vi "main 1.1 stable.vi"() -> ()   [LabVIEW 2020]
uses:
  subvi/Newport ESP301/Newport ESP301.lvlib
  subvi/sp_manip.llb/sp_manip_lib.lvlib
  subvi/sp_manip.llb/tcp_gateway.lvlib
  subvi/PHOIBOS/DEFINITIONS/DEF_dev_type.ctl
  subvi/PHOIBOS/DEFINITIONS/DEF_dev_state.ctl
  <vilib>/Utility/file.llb/Write Delimited Spreadsheet (DBL).vi
  <vilib>/Analysis/NI_AALBase.lvlib
  <vilib>/Analysis/1siggen.llb/Ramp Pattern by Samples.vi
  <vilib>/Analysis/NI_AALPro.lvlib
  <vilib>/Analysis/_algsub.llb/Real Vector Norm.vi
  subvi/ZaberTSeries/ZaberTSeries.lvlib
  <vilib>/DAQmx/create/channels.llb/DAQmx Create Channel (DI-Digital Input).vi
  <vilib>/Utility/file.llb/Read Delimited Spreadsheet (string).vi
  <vilib>/Utility/file.llb/Write Delimited Spreadsheet (string).vi
panel:
  out "Pics L":i32=20
  out "Waveform Chart":dbl(graph)
  out "G2 X":cluster{dbl[], "Ramp Pattern":dbl[]}(graph)
  in  "reset every n pics":bool=TRUE
  in  "pics2avg":i32=50
  in  "abort acq.":bool
  out "G2 Y":cluster{dbl[], "Ramp Pattern":dbl[]}(graph)={[0.0, 0.0, 0.0, 0.0, 0.0, 0.0, 0.0, 0.0, 0.0, 0.0, 0.0, 0.0, 0.0, 0.0, 0.0, 0.0, 0.0, 0.0, 0.0, 0.0, 0.0, 0.0, 0.0, 0.0, 0.0, 0.0, 0.0, 0.0, 0.0, 0.0, 0.0, 0.0, 0.0, 0.0, 0.0, 0.0, 0.0, 0.0, 0.0, 0.0, 0.0, 0.0, 0.0, 0.0, 0.0, 0.0, 0.0, 0.0, 0.0, 0.0, 0.0, 0.0, 0.0, 0.0, 0.0, 0.0, 0.0, 0.0, 0.0, 0.0, 0.0, 0.0, 0.0, 0.0, 0.0, 0.0, 0.0, 0.0, 0.0, 0.0, 0.0, 0.0, 0.0, 0.0, 0.0, 0.0, 0.0, 0.0, 0.0, 0.0, 0.0, 0.0, 0.0, 0.0, 0.0, 0.0, 0.0, 0.0, 0.0, 0.0, 0.0, 0.0, 0.0, 0.0, 0.0, 0.0, 0.0, 0.0, 0.0, 0.0, 0.0, 0.0, 0.0, 0.0, 0.0, 0.0, 0.0, 0.0, 0.0, 0.0, 0.0, 0.0, 0.0, 0.0, 0.0, 0.0, 0.0, 0.0, 0.0, 0.0, 0.0, 0.0, 0.0, 0.0, 0.0, 0.0, 0.0, 0.0, 0.0, 0.0, 0.0, 0.0, 0.0, 0.0, 0.0, 0.0, 0.0, 0.0, 0.0, 0.0, 0.0, 0.0, 0.0, 0.0, 0.0, 0.0, 0.0, 0.0, 0.0, 0.0, 0.0, 0.0, 0.0, 0.0, 0.0, 0.0, 0.0, 0.0, 0.0, 0.0, 0.0, 0.0, 0.0, 0.0, 0.0, 0.0, 0.0, 0.0, 0.0, 0.0, 0.0, 0.0, 0.0, 0.0, 0.0, 0.0, 0.0, 0.0, 0.0, 0.0, 0.0, 0.0, 0.0, 0.0, 0.0, 0.0, 0.0, 0.0, 0.0, 0.0, 0.0, 0.0, 0.0, 0.0, 0.0, 0.0, 0.0, 0.0, 0.0, 0.0, 0.0, 0.0, 0.0, 0.0, 0.0, 0.0, 0.0, 0.0, 0.0, 0.0, 0.0, 0.0, 0.0, 0.0, 0.0, 0.0, 0.0, 0.0, 0.0, 0.0, 0.0, 0.0, 0.0, 0.0, 0.0, 0.0, 0.0, 0.0, 0.0, 0.0, 0.0, 0.0, 0.0, 0.0, 0.0, 0.0, 0.0, 0.0, 0.0, 0.0, 0.0, 0.0, 0.0, 0.0, 0.0, 0.0, 0.0, 0.0, 0.0, 0.0, 0.0, 0.0, 0.0, 0.0, 0.0, 0.0], "Ramp Pattern"=[0.0, 1.003921568627451, 2.007843137254902, 3.011764705882353, 4.015686274509804, 5.019607843137255, 6.023529411764706, 7.027450980392157, 8.031372549019608, 9.035294117647059, 10.03921568627451, 11.04313725490196, 12.047058823529412, 13.050980392156863, 14.054901960784314, 15.058823529411764, 16.062745098039215, 17.066666666666666, 18.070588235294117, 19.07450980392157, 20.07843137254902, 21.08235294117647, 22.08627450980392, 23.090196078431372, 24.094117647058823, 25.098039215686274, 26.101960784313725, 27.105882352941176, 28.109803921568627, 29.113725490196078, 30.11764705882353, 31.12156862745098, 32.12549019607843, 33.129411764705885, 34.13333333333333, 35.13725490196079, 36.141176470588235, 37.14509803921569, 38.14901960784314, 39.15294117647059, 40.15686274509804, 41.16078431372549, 42.16470588235294, 43.168627450980395, 44.17254901960784, 45.1764705882353, 46.180392156862744, 47.1843137254902, 48.188235294117646, 49.1921568627451, 50.19607843137255, 51.2, 52.20392156862745, 53.207843137254905, 54.21176470588235, 55.21568627450981, 56.219607843137254, 57.22352941176471, 58.227450980392156, 59.23137254901961, 60.23529411764706, 61.23921568627451, 62.24313725490196, 63.247058823529414, 64.25098039215686, 65.25490196078431, 66.25882352941177, 67.26274509803922, 68.26666666666667, 69.27058823529411, 70.27450980392157, 71.27843137254902, 72.28235294117647, 73.28627450980392, 74.29019607843138, 75.29411764705883, 76.29803921568627, 77.30196078431372, 78.30588235294118, 79.30980392156863, 80.31372549019608, 81.31764705882352, 82.32156862745099, 83.32549019607843, 84.32941176470588, 85.33333333333333, 86.33725490196079, 87.34117647058824, 88.34509803921569, 89.34901960784313, 90.3529411764706, 91.35686274509804, 92.36078431372549, 93.36470588235294, 94.3686274509804, 95.37254901960785, 96.37647058823529, 97.38039215686274, 98.3843137254902, 99.38823529411765, 100.3921568627451, 101.39607843137254, 102.4, 103.40392156862745, 104.4078431372549, 105.41176470588235, 106.41568627450981, 107.41960784313726, 108.4235294117647, 109.42745098039215, 110.43137254901961, 111.43529411764706, 112.43921568627451, 113.44313725490196, 114.44705882352942, 115.45098039215686, 116.45490196078431, 117.45882352941176, 118.46274509803922, 119.46666666666667, 120.47058823529412, 121.47450980392156, 122.47843137254903, 123.48235294117647, 124.48627450980392, 125.49019607843137, 126.49411764705883, 127.49803921568628, 128.50196078431372, 129.50588235294117, 130.50980392156862, 131.51372549019607, 132.51764705882354, 133.521568627451, 134.52549019607844, 135.52941176470588, 136.53333333333333, 137.53725490196078, 138.54117647058823, 139.54509803921567, 140.54901960784315, 141.5529411764706, 142.55686274509804, 143.5607843137255, 144.56470588235294, 145.5686274509804, 146.57254901960783, 147.57647058823528, 148.58039215686276, 149.5843137254902, 150.58823529411765, 151.5921568627451, 152.59607843137255, 153.6, 154.60392156862744, 155.6078431372549, 156.61176470588236, 157.6156862745098, 158.61960784313726, 159.6235294117647, 160.62745098039215, 161.6313725490196, 162.63529411764705, 163.6392156862745, 164.64313725490197, 165.64705882352942, 166.65098039215687, 167.65490196078431, 168.65882352941176, 169.6627450980392, 170.66666666666666, 171.6705882352941, 172.67450980392158, 173.67843137254903, 174.68235294117648, 175.68627450980392, 176.69019607843137, 177.69411764705882, 178.69803921568626, 179.7019607843137, 180.7058823529412, 181.70980392156864, 182.71372549019608, 183.71764705882353, 184.72156862745098, 185.72549019607843, 186.72941176470587, 187.73333333333332, 188.7372549019608, 189.74117647058824, 190.7450980392157, 191.74901960784314, 192.75294117647059, 193.75686274509803, 194.76078431372548, 195.76470588235293, 196.7686274509804, 197.77254901960785, 198.7764705882353, 199.78039215686275, 200.7843137254902, 201.78823529411764, 202.7921568627451, 203.79607843137254, 204.8, 205.80392156862746, 206.8078431372549, 207.81176470588235, 208.8156862745098, 209.81960784313725, 210.8235294117647, 211.82745098039214, 212.83137254901962, 213.83529411764707, 214.8392156862745, 215.84313725490196, 216.8470588235294, 217.85098039215686, 218.8549019607843, 219.85882352941175, 220.86274509803923, 221.86666666666667, 222.87058823529412, 223.87450980392157, 224.87843137254902, 225.88235294117646, 226.8862745098039, 227.89019607843136, 228.89411764705883, 229.89803921568628, 230.90196078431373, 231.90588235294118, 232.90980392156862, 233.91372549019607, 234.91764705882352, 235.92156862745097, 236.92549019607844, 237.9294117647059, 238.93333333333334, 239.93725490196078, 240.94117647058823, 241.94509803921568, 242.94901960784313, 243.95294117647057, 244.95686274509805, 245.9607843137255, 246.96470588235294, 247.9686274509804, 248.97254901960784, 249.9764705882353, 250.98039215686273, 251.98431372549018, 252.98823529411766, 253.9921568627451, 254.99607843137255, 256.0]}
  out "ETA":timestamp=timestamp(3553173084.423481 s since 1904-01-01) format="%<%H:%M:%S>T"
  out "acq. imgs":i32=20
  out "snap_prog":dbl(slide)=1.0 scale=0.0..1.0
  in  "BasePath":path=path "Z:/PESdata"
  in  "cam_liveavg":bool=TRUE caption="live average"
  out "cam_fps":dbl=19.770971874875205 caption="FPS" format="%.1g"
  out "sideimg":dbl[][](graph)
  out "RunNumber":u16=50
  out "sum":dbl format="%#.2g"
  out "max":dbl
  out "mainimg":dbl[][](graph)
  out "ESP_con?":bool=TRUE caption="ESP301"
  out "phoib_con?":bool caption="PHOIBOS"
  out "manip_con?":bool=TRUE caption="manipulator"
  out "cam_con?":bool caption="camera"
  in  "main_close":bool
  in  "Tab Control":enum32{"live", "1D scan", "devices"}(tab)=enum."1D scan"
  in  "mirr_go":bool
  in  "ESP_opent0file":bool
  in  "mirr_rel":i32=20 caption="relative [steps]"
  in  "mirr_Y-":bool
  in  "mirr_Y+":bool
  in  "mirr_X+":bool
  in  "mirr_X-":bool
  in  "manip_deltas":dbl[](array[numeric])=[0.0, 0.0, 5.0, 0.0, 0.0, 0.0] caption="delta" format="%#.5g"
  in  "aq.mode":enum32{"Radio Selection 1", "Radio Selection 2"}(radio)=enum."Radio Selection 2"
  in  "dark avg":i32=100
  in  "cam_avgs":i32=20 caption="N"
  in  "ESP_delta":dbl caption="relative [mm]"
  in  "ESP_-":bool
  in  "ESP_+":bool
  in  "ESP_go":bool
  in  "ESP_dest_t":dbl=-12656.75602819869 caption="[fs]"
  in  "ESP_dest":dbl=25.0 caption="[mm]"
  in  "ESP_set_t0":bool
  in  "phoib_I_6s":dbl=3200.0
  in  "phoib_I_5s":dbl=1500.0
  in  "phoib_I_4s":dbl=4.558
  in  "phoib_I_3s":dbl=-7.0
  in  "phoib_I_2s":dbl=30.0
  in  "phoib_I_1s":dbl=18.0
  in  "phoib_standby":bool
  in  "phoib_set":bool
  out "phoib_I_6":dbl caption="Screen Voltage"
  out "phoib_I_5":dbl caption="Detctor Voltage"
  out "phoib_I_4":dbl caption="Work Function"
  out "phoib_I_3":dbl caption="Coil Current"
  out "phoib_I_2":dbl caption="Pass Energy"
  out "phoib_I_1":dbl caption="Kinetic Energy"
  out "Saved Positions":string[][](table)=[["ertwertwert", "-2.299945", "-2.030214", "38.900024", "50.000762", "0.000887", "-97.998082"], ["uztgugt", "-14.999451", "-13.638894", "442.380066", "13.998380", "-1.893758", "-76.305838"], ["asdf", "-14.999451", "-13.638894", "442.380066", "13.998380", "-1.893758", "-76.305838"], ["test3", "-14.999451", "-13.638894", "441.380066", "13.998380", "-1.893758", "-76.305838"]]
  in  "Save Pos":bool
  in  "Load":bool
  in  "Delete":bool
  in  "ManipRel +":bool
  in  "ManipRel -":bool
  in  "Move Abs":bool
  in  "stop manip":bool
  in  "dest":dbl[](array[numeric])=[-2.599774415331921, 2.6001372083008483, 64.7374267578125, 44.999124169862, 0.0008789063100814859, -80.99718876558107] caption="destination" format="%#.5g"
  out "axis":string[](array[string])=["x", "y", "z", "polar", "tilt", "azimut"]
  out "pos":dbl[](array[numeric])=[-1.8981328134268227, 1.9037561044451934, 84.7381591796875, 38.14189713860625, 0.0008789063100814859, -70.9987511093555] caption="position" format="%.5f"
  in  "ana_mode":T1(ring)=enum."WideAngleMode"
  in  "ana_voltrange":enum16{"3.5kV", "1.5kV", "400V", "100V", "10V"}(ring)=enum."400V"
  out "ESP_pos":dbl=31.74535 caption="Position"
  out "ESP_delay":dbl=45000.131390897084 caption="Delay"
  out "ESP_t0":dbl=25.0 caption="Time Zero @"
  out "phoib_I_7":dbl caption="Conversion Voltage"
  in  "phoib_I_7s":dbl=-26.0
  in  "phoib_I_8s":dbl=0.0039
  in  "phoib_I_9s":dbl=0.0039
  out "phoib_I_8":dbl caption="FD1"
  out "phoib_I_9":dbl caption="FD2"
  in  "gain":bool
  in  "cam_exp":u32=50 caption="exposure [ms]"
  in  "binning":u16(ring)=2 items=["X 1", "X 2", "X 4", "X 8"]
  in  "cam_dark?":bool=TRUE caption="subtract dark?"
  in  "cam_dark":bool
  in  "cam_saveimg":bool
  in  "e-size":u8
  in  "lower threshold":i32=50
  in  "count?":bool
  in  "ROI Left":i32=1
  in  "ROI Right":i32=43
  in  "ROI Top":i32=1
  in  "ROI Bottom":i32=33
  out "moving?":bool[](array[boolean])
  out "mirr_posX":i32=-9907 caption="X"
  out "mirr_posY":i32=-7260 caption="Y"
  in  "mirr_dest":i32[](array[numeric])=[-64, -2601]
  out "anglegraph":dbl[][](graph)
  out "intensitygraph":cluster{"Array":dbl[], "Intensity Chart":dbl[]}(graph)={"Array"=[-100000.0, -95000.0, -90000.0, -85000.0, -80000.0, -75000.0, -70000.0, -65000.0, -60000.0, -55000.0, -50000.0, -45000.0, -40000.0, -35000.0, -30000.0, -25000.0, -20000.0, -15000.0, -10000.0, -5000.0, 0.0, 5000.0, 10000.0, 15000.0, 20000.0, 25000.0, 30000.0, 35000.0, 40000.0, 45000.0, 50000.0], "Intensity Chart"=[710968.0999999978, 661453.8299999974, 660491.1499999983, 654490.9100000008, 607000.039999999, 668861.0999999981, 631366.7699999984, 739689.6549999982, 681310.9099999986, 658872.4599999987, 692812.8950000014, 671304.7250000003, 670701.9799999978, 684100.4049999971, 706126.3150000001, 744782.0600000009, 684440.8499999981, 704157.155, 756957.4599999988, 768506.4449999956, 761428.5800000022, 678039.9949999974, 735774.9649999988, 659533.465000001, 724648.9199999974, 705546.0750000002, 773026.2399999972, 698578.0149999986, 697856.3899999985, 787613.0450000013, 750231.4800000007]}
  in  "scan_selector":enum32{"delay", "manip", "mirror", "volt"}(tab)
  in  "scan_manip_setstart":bool
  in  "scan_manip_start":dbl[](array[numeric])=[-2.6172862113166087, -0.009888298846365134, 68.5008544921875, -46.363686276590336, 11.108982061941884, -218.56360350415366] caption="start position" format="%#.5g"
  in  "scan_manip_deltas":dbl[](array[numeric])=[0.0, 0.0, 0.0, 0.0, 10.0, 0.0] caption="direction vector\n(gets normed)" format="%#.5g"
  in  "scan_mirr_start":i32[](array[numeric])=[-64, -2601]
  in  "scan_mirr_deltas":i32[](array[numeric])=[0, 0, 0, 0, 10, 0] caption="direction vector\n(gets normed)"
  in  "scan_mirr_setstart":bool
  in  "scan_volt_parameter":string(combo)="Kinetic Energy"
  in  "meas_iter":i32=60 caption="Iterations"
  out "duration [HH:MM:SS]":dbl=4512.494100093842 format="%<%H:%M:%S>t"
  out "disk [MB]":dbl=1028.5800000000002
  out "RAM [MB]":dbl=17.143
  out "total steps":i32=1860
  out "measpoints":i32=31
  in  "load delay table":bool
  in  "scan_go":bool
  in  "waypoints":string[][](table)=[["-100000", "5000"], ["50000", ""], ["", ""]]
  in  "stop after step":bool
  out "scan":dbl(slide)=0.967741935483871 scale=0.0..1.0
  out "iteration":dbl(slide)=0.03333333333333333 scale=0.0..1.0
  out "current scan":i32=30
  out "current iteration":i32=2
  in  "time/step [s]":dbl=2.426072096824646
  in  "stop after iteration":bool
  out "energygraph":dbl[][](graph)
  in  "mirr_init":bool
  in  "mirr_release":bool
  in  "mirr_Y#":u8=2
  in  "manip_init":bool
  in  "manip_release":bool
  in  "phoib_init":bool
  in  "phoib_release":bool
  in  "ESP_init":bool
  in  "ESP_release":bool
  in  "ESP301 VISA":refnum<visa-resource-name>="COM8"
  in  "board number":i32
  in  "cam_init":bool
  in  "cam_release":bool
  out "cam_error":errorcluster
  out "phoib_error":errorcluster
  out "state":T2 items=["Off"=-1, "Standby"=0, "On"=1]
  in  "ESP Axis":i32=1 min=1 max=3
  out "error out":errorcluster
  out "error out 2":errorcluster
  out "mirr_Error":errorcluster
  in  "mirr_VISA":refnum<visa-resource-name>="COM7"
  in  "mirr_X#":u8=1
  in  "Operating mode\nHP & QE / HS & DiCam Pro":u32=1
  in  "Frame trigger \n(High Performance and QE only)":u16
  # "camera"
  # "analyzer"
  # "manipulator"
  # "aquisition"
  # "delay stage"
  # "mirror"
  # "Position"
  # "Destination"
  # "- no settings -"
  # "waypoints are absolute values"
  # "X\nY\nZ\npolar\ntilt\nazimut"
  # "waypoint \"0\" is start position"
  # "X\nY"
  # "waypoint \"0\" is start position"
  # "waypoints are absolute values"
  # "camera"
  # "phoibos"
  # "ESP301"
  # "manipulator"
  # "mirror"
  # "0 = sequential\n1 = simultaneous"
  # "0 = internal\n1 = external rising\n2 = external falling"
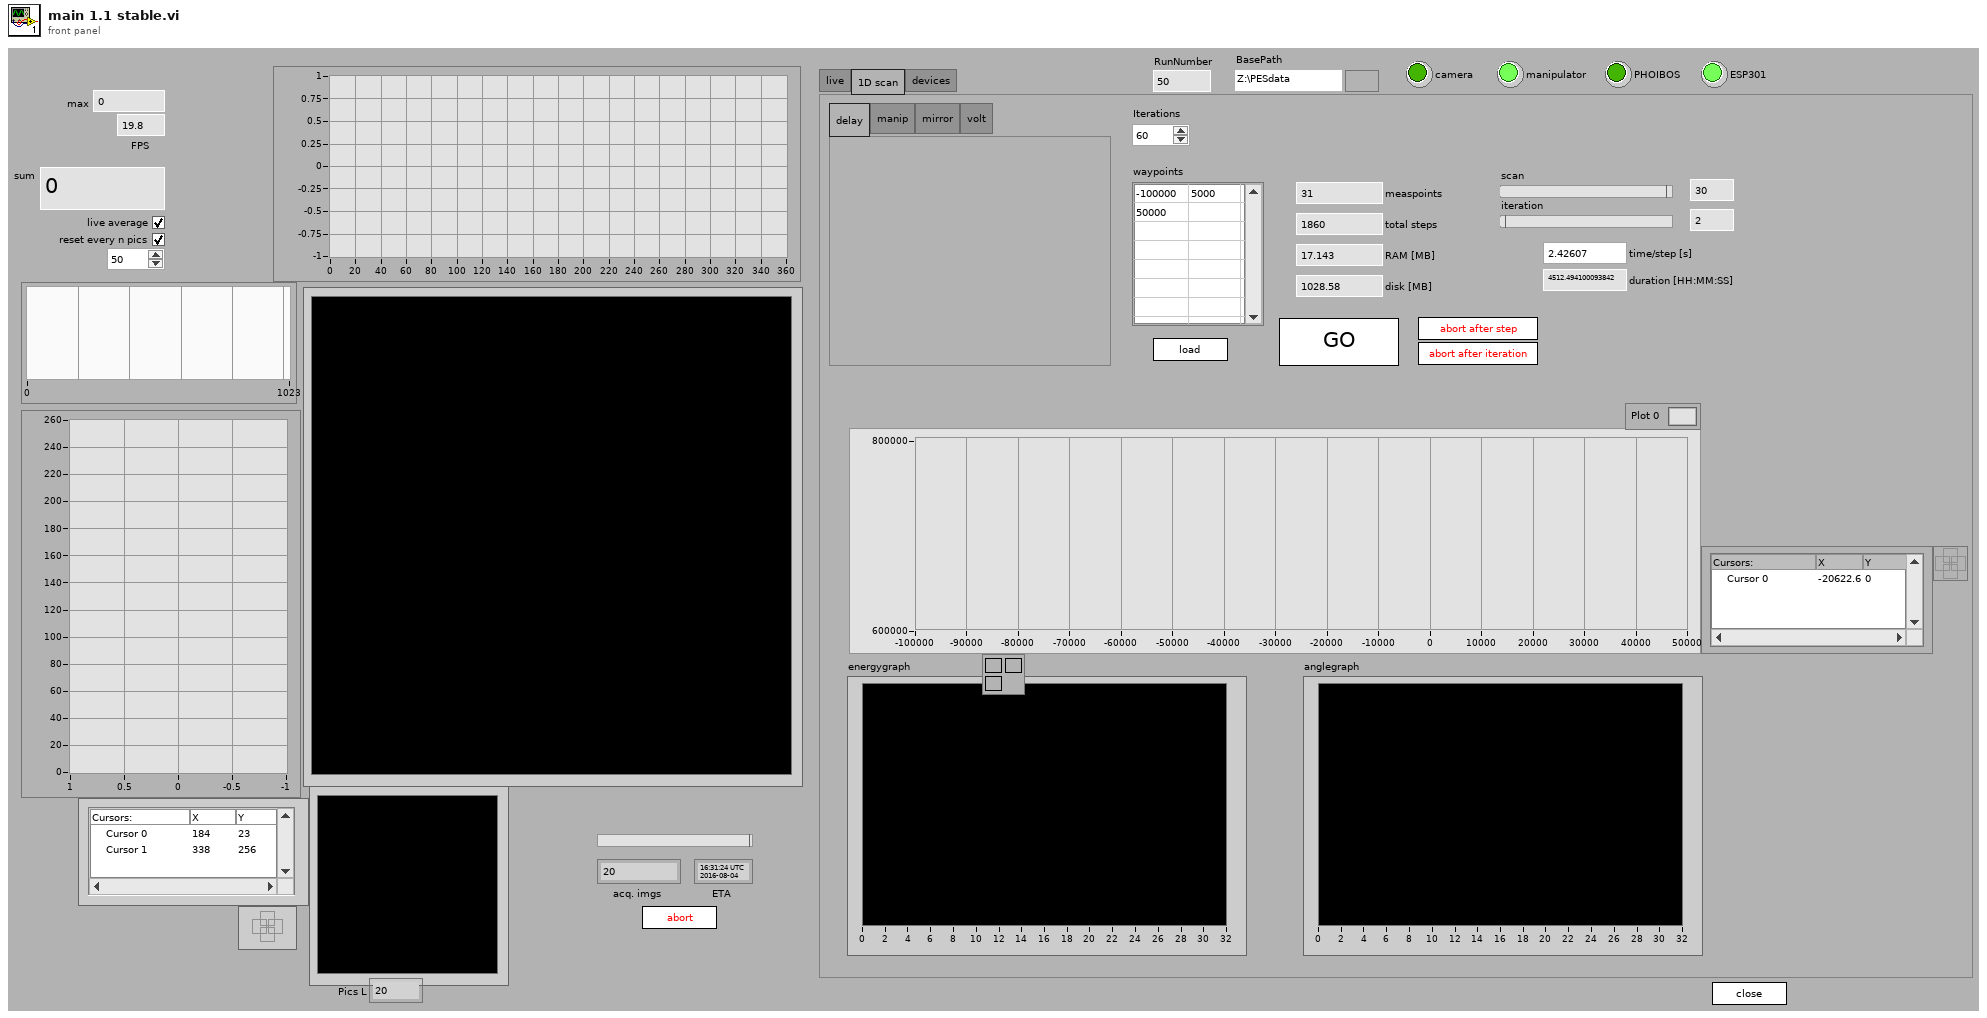
[diagram p1: front panel]
types:
  T1 = enum16{"HighMagnification", "MediumMagnification", "LowMagnification", "HighAngularDispersion", "MediumAngularDispersion", "LowAngularDispersion", "WideAngleMode", "LargeArea", "MediumArea", "SmallArea", "HighMagnification2", "SmallArea2", "ImagingMode"}
  T2 = typedef "DEF_dev_state.ctl" = i32
  T3 = cluster{"queue out":refnum<queue>, "queue out":refnum<queue>, "queue out":refnum<queue>, "queue out":refnum<queue>, "queue out":refnum<queue>}
  T4 = typedef "LVCursorListTypeDef.ctl" = cluster{"Name":string, "Color":u32, "Style":u8, "Point Style":u8, "Name Visible":bool, "Allow Drag":bool, "Cursor Mode":u32, "Plot":i32, "Index":i32, "Position":cluster{"X":dbl, "Y":dbl}, "X Scale":u32, "Y Scale":u32, "Watch Plots":i32[], "Watch All Plots":bool, "Plot Area":i32, "Label Offset":cluster{"X":dbl, "Y":dbl}}[]
  T5 = cluster{"Camera type":u32, "Operating mode\nHP & QE / HS & DiCam Pro ":u32, "Frame trigger \n(High Performance and QE only)":u16, "Sequence trigger":u16, "Low Light\n(QE only)":bool, "Gain":bool, "Horzontal\nbinning":u16, "Vertical\nbinning ":u16, "ROI Left":i32, "ROI Right":i32, "ROI Top":i32, "ROI Bottom":i32}
  T6 = cluster{"Name":string, "Color":u32, "Style":u8, "Point Style":u8, "Name Visible":bool, "Allow Drag":bool, "Cursor Mode":u32, "Plot":i32, "Index":i32, "Position":cluster{"X":dbl, "Y":dbl}, "X Scale":u32, "Y Scale":u32, "Watch Plots":i32[], "Watch All Plots":bool, "Plot Area":i32, "Label Offset":cluster{"X":dbl, "Y":dbl}}
  T7 = cluster{"mirr_X#":u8, "Command":u8, dbl, "Response Count":i32}
  T8 = cluster{"mirr_Y#":u8, "Command":u8, dbl, "Response Count":i32}
  T9 = cluster{i32, "Command":u8, i32, "Response Count":i32}
  T10 = cluster{"Axis_Name":string, "Axis_Type":string, "Axis_Position":dbl, "continous":bool, "moving":bool}[]
  T11 = typedef "DEF_dev_type.ctl" = enum32{"devA (analyzer)", "devD (detector)"}
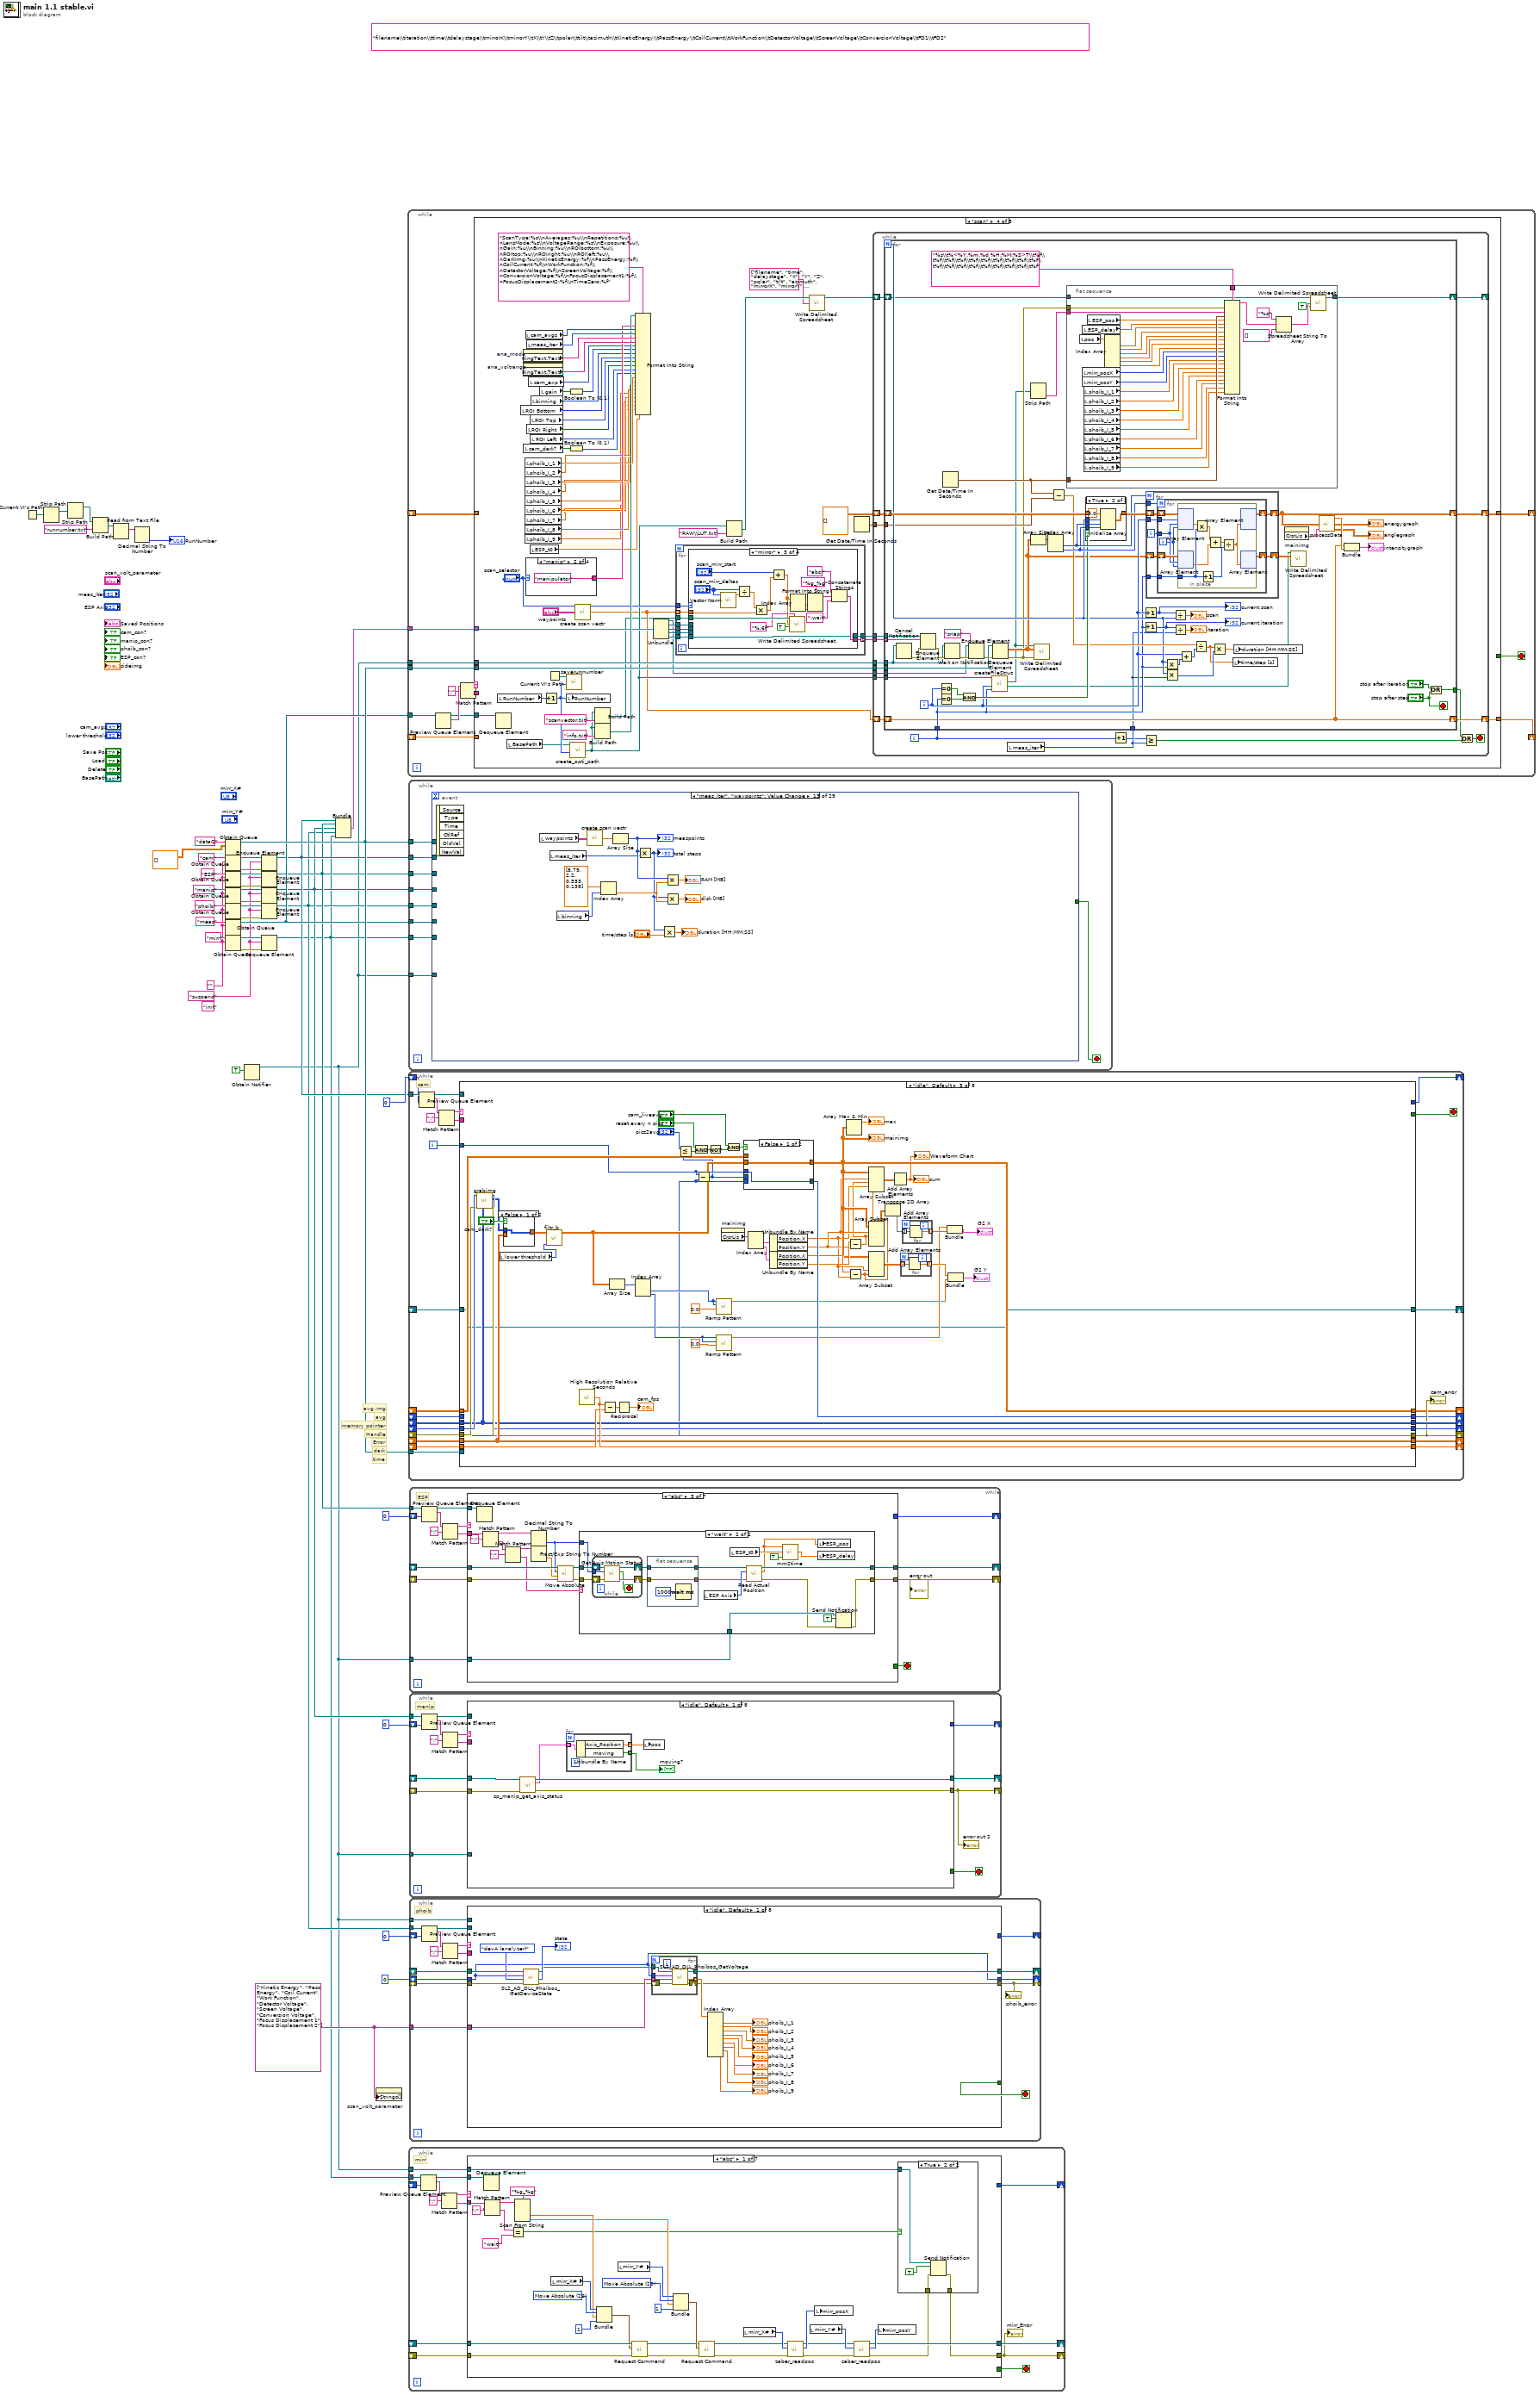
[diagram p0: block diagram]
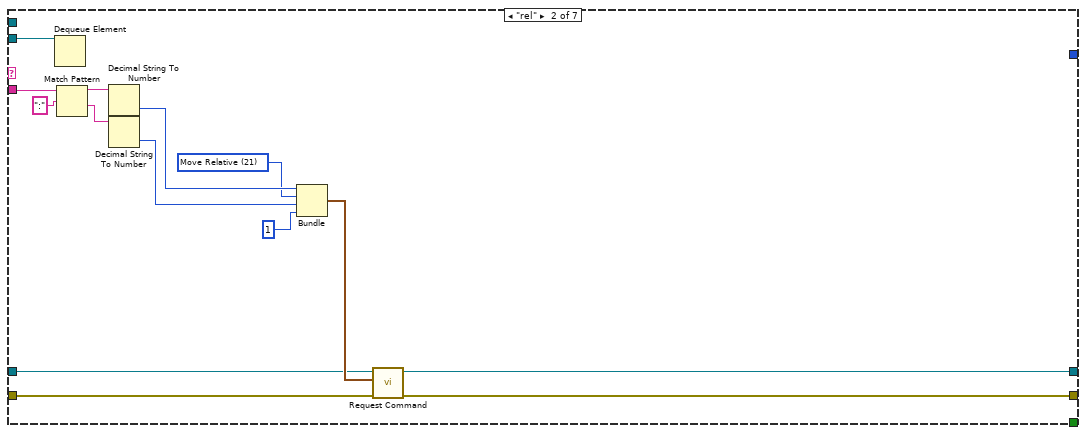
[diagram p3: hidden frame]
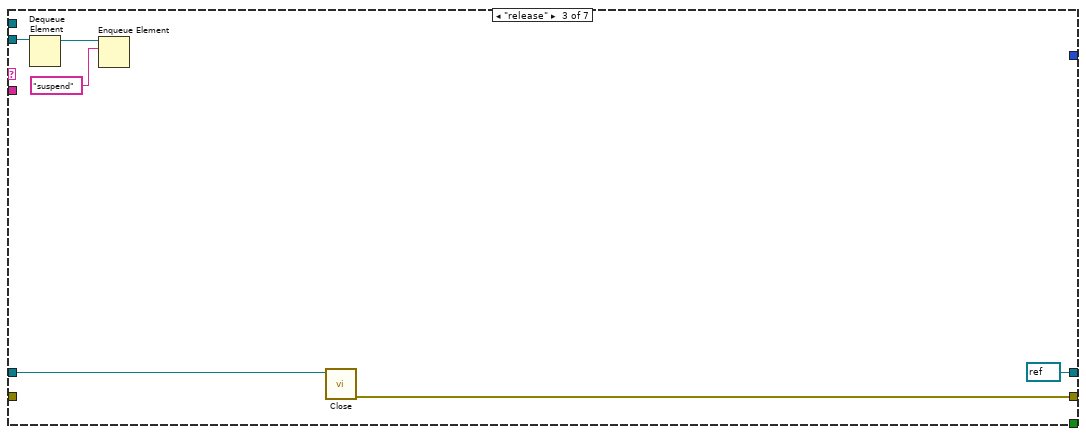
[diagram p4: hidden frame]
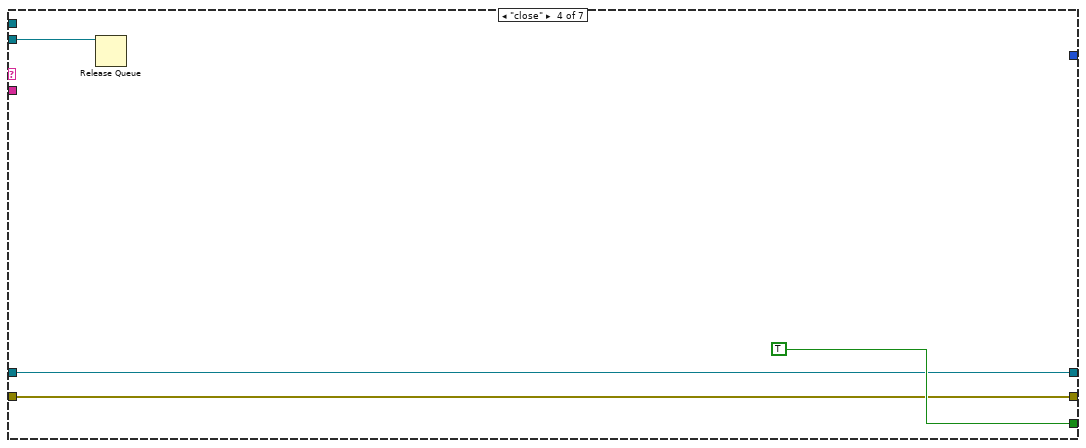
[diagram p5: hidden frame]
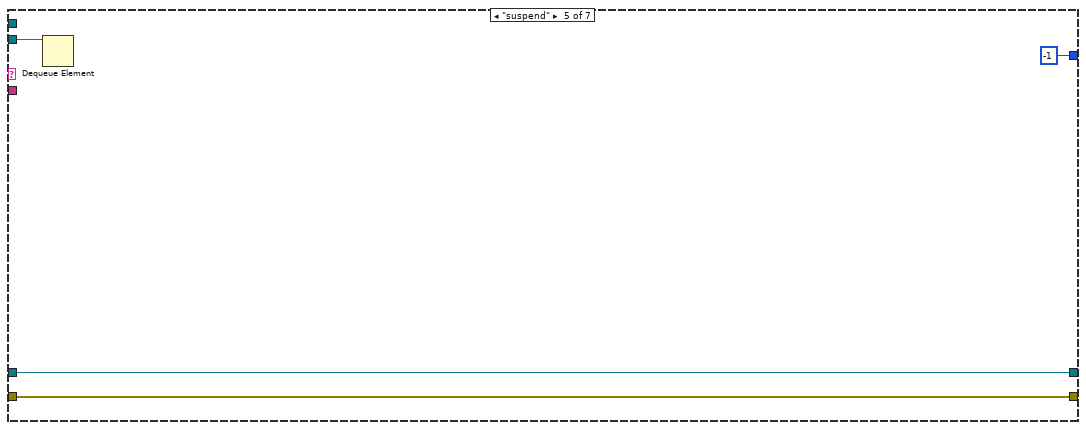
[diagram p6: hidden frame]
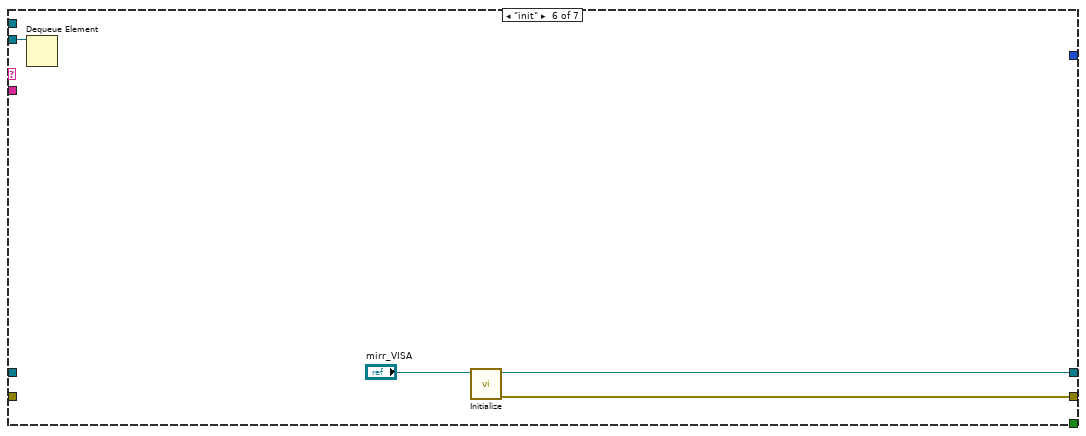
[diagram p7: hidden frame]
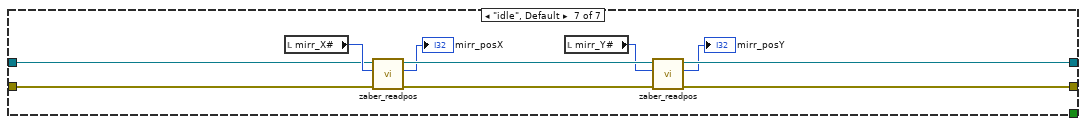
[diagram p8: hidden frame]
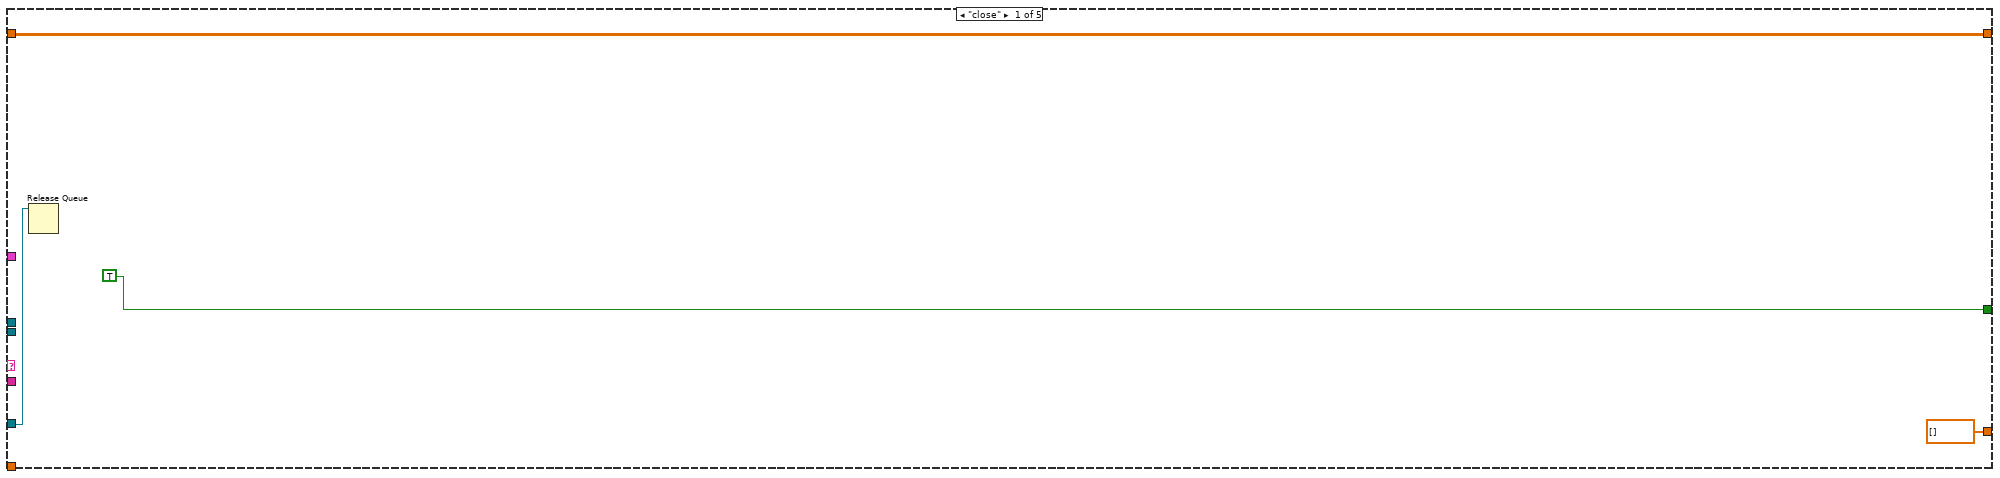
[diagram p9: hidden frame]
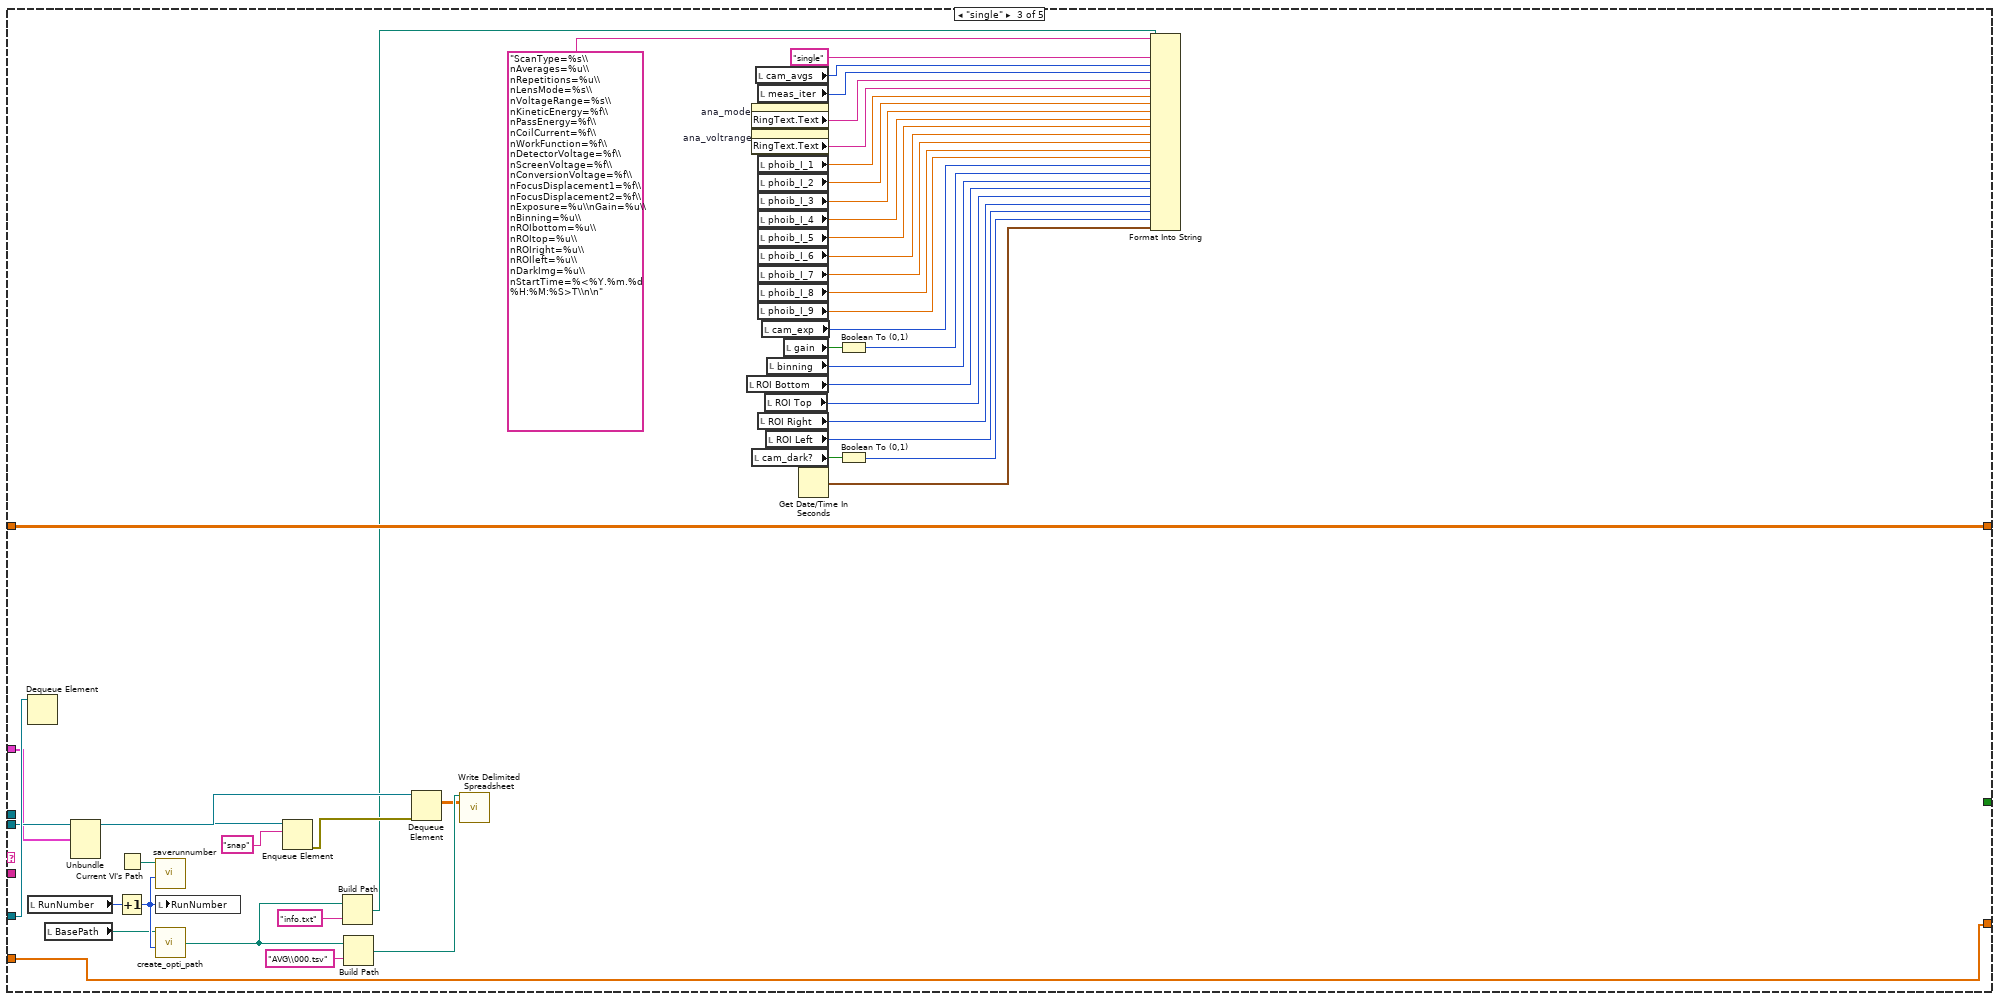
[diagram p11: hidden frame]
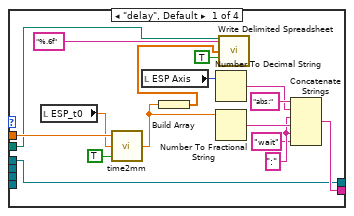
[diagram p13: hidden frame]
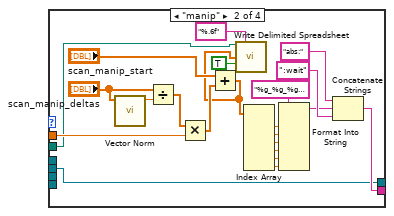
[diagram p14: hidden frame]
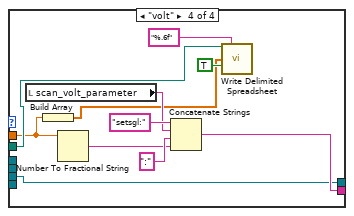
[diagram p15: hidden frame]
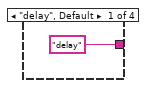
[diagram p16: hidden frame]
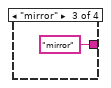
[diagram p17: hidden frame]
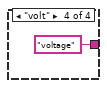
[diagram p18: hidden frame]
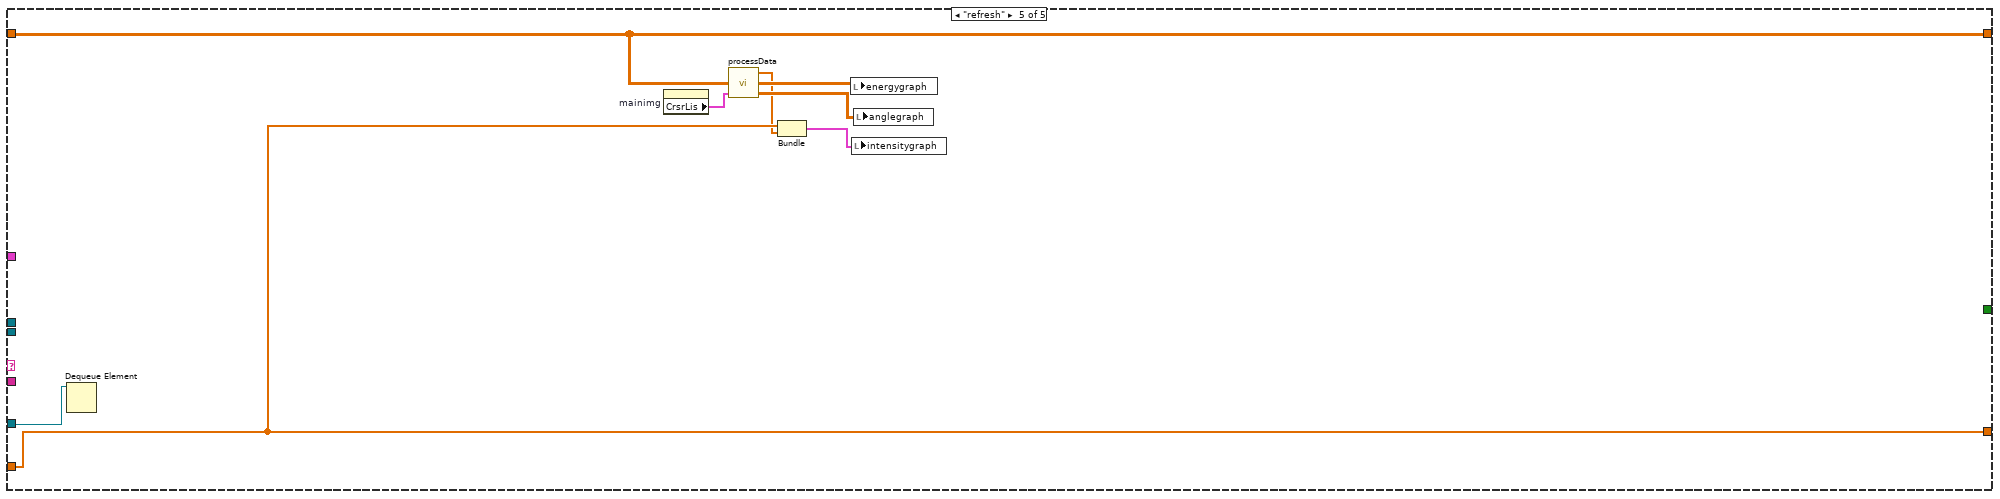
[diagram p19: hidden frame]
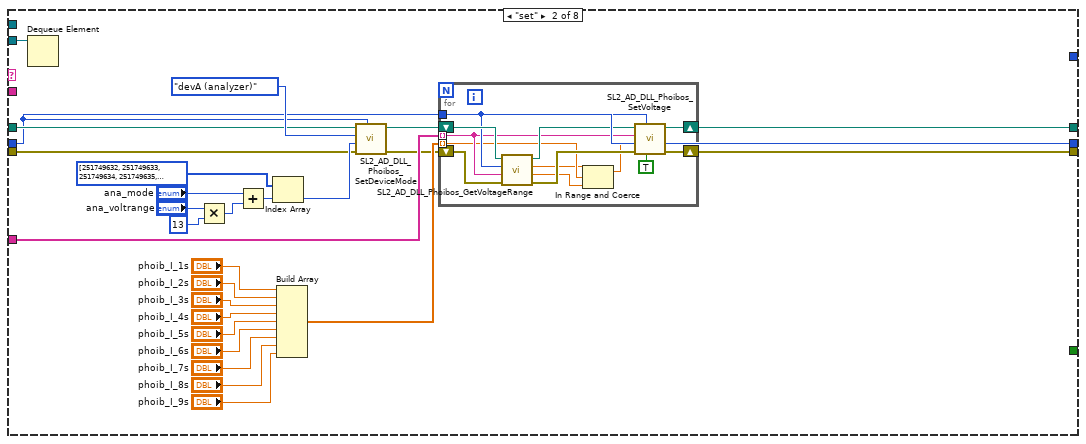
[diagram p20: hidden frame]
diagram:
  (unwired) "filename\\titeration\\ttime\\tdelaystage\\tmirrorX\\tmirrorY\\tX\\tY\\tZ\\tpolar\\ttilt\\tazimuth\\tKineticEnergy\\tPassEnergy\\tCoilCurrent\\tWorkFunction\\tDetectorVoltage\\tScreenVoltage\\tConversionVoltage\\tFD1\\tFD2"
  w9 = string[] ["Kinetic Energy", "Pass Energy", "Coil Current", "Work Function", "Detector Voltage", "Screen Voltage", "Conversion Voltage", "Focus Displacement 1", "Focus Displacement 2"]
  (unwired) "init" ("name (unnamed)")
  w1 = "suspend" ("name (unnamed)")
  w2 = "" ("name (unnamed)")
  # "avg img"
  # "avg"
  # "time"
  # "dark"
  # "Error"
  # "Handle"
  # "memory pointer"
  n1 = Current VI's Path() -> (path=w17:path)
  n2 = Strip Path(path=w17) -> (stripped path=w21:path)  [unwired: 1 out]
  n3 = Strip Path(path=w21) -> (stripped path=w22:path)  [unwired: 1 out]
  n4 = Build Path(base path=w22, name or relative path="runnumber.txt") -> (appended path=w19:path)
  n5 = Read from Text File(file (use dialog)=w19) -> (text=w20:string)  [unwired: 3 in, 3 out]
  n6 = Decimal String To Number(string=w20) -> (number=→"RunNumber":i32)  [unwired: 2 in, 1 out]
  n7 = Obtain Queue(name (unnamed)="dataQ", element data type=dbl[][] []) -> (queue out=w23:refnum<queue>)  [unwired: 3 in, 2 out]
  n8 = Obtain Queue(name (unnamed)="cam", element data type=w2) -> (queue out=w42:refnum<queue>, error out=w41:errorcluster)  [unwired: 3 in, 1 out]
  n9 = Obtain Queue(name (unnamed)="ESP", element data type=w2) -> (queue out=w39:refnum<queue>, error out=w40:errorcluster)  [unwired: 3 in, 1 out]
  n10 = Obtain Queue(name (unnamed)="manip", element data type=w2) -> (queue out=w36:refnum<queue>, error out=w35:errorcluster)  [unwired: 3 in, 1 out]
  n11 = Obtain Queue(name (unnamed)="phoib", element data type=w2) -> (queue out=w33:refnum<queue>, error out=w34:errorcluster)  [unwired: 3 in, 1 out]
  n12 = Obtain Queue(name (unnamed)="meas", element data type=w2) -> (queue out=w16:refnum<queue>)  [unwired: 3 in, 2 out]
  n13 = Obtain Queue(name (unnamed)="mirr", element data type=w2) -> (queue out=w7:refnum<queue>, error out=w6:errorcluster)  [unwired: 3 in, 1 out]
  n14 = Obtain Notifier(notification data type=TRUE) -> (notifier out=w3:refnum<notifier>)  [unwired: 3 in, 2 out]
  n15 = Enqueue Element(queue=w42, element=w1, error in (no error)=w41) -> (queue out=w14:refnum<queue>)  [unwired: 1 in, 2 out]
  n16 = Enqueue Element(queue=w39, element=w1, error in (no error)=w40) -> (queue out=w13:refnum<queue>)  [unwired: 1 in, 2 out]
  n17 = Enqueue Element(queue=w36, element=w1, error in (no error)=w35) -> (queue out=w12:refnum<queue>)  [unwired: 1 in, 2 out]
  n18 = Enqueue Element(queue=w33, element=w1, error in (no error)=w34) -> (queue out=w11:refnum<queue>)  [unwired: 1 in, 2 out]
  n19 = Enqueue Element(queue=w7, element=w1, error in (no error)=w6) -> (queue out=w4:refnum<queue>)  [unwired: 1 in, 2 out]
  n20 = Bundle("queue out"=w14, "queue out"=w13, "queue out"=w12, "queue out"=w11, "queue out"=w4) -> (w15:T3)  [unwired: 1 in]
  n21 = property on="scan_volt_parameter" class="CmbBox"("Strings[]"=w9) -> ()  [unwired: 2 in, 2 out]
  n22 = while {
    tunnel: w23 -> [w57]
    tunnel: w16 -> [w54]
    tunnel: w15 -> [w50]
    shift-right: [w48] -> _
    shift-left: _ -> [w47]
    tunnel: w3 -> [w46]
    shift-right: [w45] -> _
    shift-left: _ -> [w44]
    stop <- w49 stop-if-true
    n23 = Preview Queue Element(queue=w54) -> (queue out=w51:refnum<queue>, element=w56:string)  [unwired: 2 in, 2 out]
    n24 = Match Pattern(string=w56, regular expression=":") -> (before substring=w53:string, after substring=w52:string)  [unwired: 1 in, 2 out]
    n25 = case shown="\"scan\"" w53 {
      tunnel: w57 -> [_ _ w106 w158 _]
      tunnel: w52 -> [_ _ _ _ _]
      tunnel: w51 -> [w61 _ w107 w154 w378]
      tunnel: [TRUE _ _ _ _] -> w49
      tunnel: w50 -> [_ _ w94 w134 _]
      tunnel: [w59 w63 w92 w156 w384] -> w48
      tunnel: w47 -> [w59 w63 w92 _ w384]
      tunnel: w46 -> [_ _ _ w155 _]
      tunnel: [dbl[] [] ("Array") w62 w64 w120 w380] -> w45
      tunnel: w44 -> [_ w62 w64 _ w380]
      frame "close" {
        n26 = Release Queue(queue=w61) -> ()  [unwired: 2 in, 3 out]
      }
      frame "idle", Default {
      }
      frame "single" {
        n27 = Dequeue Element(queue=w107) -> ()  [unwired: 2 in, 4 out]
        n28 = local read "RunNumber"() -> (w101:u16)
        n29 = local read "BasePath"() -> (w102:path)
        n30 = Unbundle(w94) -> ("queue out"=w93:refnum<queue>)  [unwired: 4 out]
        n31 = Increment(x=w101) -> (x+1=w103:u16)
        n32 = Current VI's Path() -> (path=w100:path)
        n33 = call "saverunnumber.vi"("RunNumber"=w103, "VI path"=w100) -> ()  [unwired: 10 in]
        n34 = local write "RunNumber"(w103) -> ()
        n35 = call "create_opti_path.vi"("RunNumber"=w103, "base path"=w102) -> ("Path"=w96:path)  [unwired: 2 in]
        n36 = Enqueue Element(queue=w93, element="snap" ("string")) -> (error out=w104:errorcluster)  [unwired: 2 in, 2 out]
        n37 = Build Path(base path=w96, name or relative path="info.txt") -> (appended path=w65:path)
        n38 = Build Path(base path=w96, name or relative path="AVG\\000.tsv") -> (appended path=w98:path)
        n39 = Dequeue Element(queue=w106, error in (no error)=w104) -> (element=w95:dbl[][])  [unwired: 1 in, 3 out]
        n40 = call-poly <vilib>:"Write Delimited Spreadsheet.vi"("file path (dialog if empty)"=w98, "2D data"=w95) -> ()  [unwired: 12 in, 2 out]
        n41 = local read "ROI Bottom"() -> (w72:i32)
        n42 = property on="ana_mode" class="Enum (strict)"() -> ("RingText.Text"=w87:string)  [unwired: 2 in, 2 out]
        n43 = property on="ana_voltrange" class="Enum (strict)"() -> ("RingText.Text"=w86:string)  [unwired: 2 in, 2 out]
        n44 = local read "cam_dark?"() -> (w68:bool)
        n45 = local read "cam_avgs"() -> (w89:i32)
        n46 = local read "meas_iter"() -> (w88:i32)
        n47 = local read "phoib_I_1"() -> (w85:dbl)
        n48 = local read "phoib_I_2"() -> (w84:dbl)
        n49 = local read "phoib_I_3"() -> (w83:dbl)
        n50 = local read "phoib_I_4"() -> (w82:dbl)
        n51 = local read "phoib_I_5"() -> (w81:dbl)
        n52 = local read "phoib_I_6"() -> (w80:dbl)
        n53 = local read "phoib_I_7"() -> (w79:dbl)
        n54 = local read "phoib_I_8"() -> (w78:dbl)
        n55 = local read "phoib_I_9"() -> (w77:dbl)
        n56 = local read "ROI Right"() -> (w70:i32)
        n57 = local read "cam_exp"() -> (w76:u32)
        n58 = local read "ROI Top"() -> (w71:i32)
        n59 = local read "ROI Left"() -> (w69:i32)
        n60 = local read "binning"() -> (w73:u16)
        n61 = local read "gain"() -> (w75:bool)
        n62 = Get Date/Time In Seconds() -> (seconds since 1Jan1904=w66:timestamp)
        n63 = Boolean To (0,1)(Boolean=w75) -> (0, 1=w74:i16)
        n64 = Boolean To (0,1)(Boolean=w68) -> (0, 1=w67:i16)
        n65 = Format Into String(format string="ScanType=%s\\nAverages=%u\\nRepetitions=%u\\nLensMode=%s\\nVoltageRange=%s\\nKineticEnergy=%f\\nPassEnergy=%f\\nCoilCurrent=%f\\nWorkFunction=%f\\nDetectorVoltage=%f\\nScreenVoltage=%f\\nConversionVoltage=%f\\nFocusDisplacement1=%f\\nFocusDisplacement2=%f\\nExposure=%u\\nGain=%u\\nBinning=%u\\nROIbottom=%u\\nROItop=%u\\nROIright=%u\\nROIleft=%u\\nDarkImg=%u\\nStartTime=%<%Y.%m.%d %H:%M:%S>T\\n\n", initial string=w65, "single" ("input 1"), w89, w88, w87, w86, w85, w84, w83, w82, w81, w80, w79, w78, w77, w76, w74, w73, w72, w71, w70, w69, w67, w66) -> ()  [unwired: 1 in, 2 out]
      }
      frame "scan" {
        n66 = Dequeue Element(queue=w154) -> ()  [unwired: 2 in, 4 out]
        n67 = local read "RunNumber"() -> (w162:u16)
        n68 = local read "BasePath"() -> (w163:path)
        n69 = local read "ROI Bottom"() -> (w140:i32)
        n70 = property on="ana_mode" class="Enum (strict)"() -> ("RingText.Text"=w149:string)  [unwired: 2 in, 2 out]
        n71 = property on="ana_voltrange" class="Enum (strict)"() -> ("RingText.Text"=w148:string)  [unwired: 2 in, 2 out]
        n72 = local read "cam_dark?"() -> (w146:bool)
        n73 = local read "phoib_I_1"() -> (w118:dbl)
        n74 = local read "phoib_I_2"() -> (w117:dbl)
        n75 = local read "phoib_I_3"() -> (w116:dbl)
        n76 = local read "phoib_I_4"() -> (w115:dbl)
        n77 = local read "phoib_I_5"() -> (w114:dbl)
        n78 = local read "phoib_I_6"() -> (w113:dbl)
        n79 = local read "phoib_I_7"() -> (w112:dbl)
        n80 = local read "phoib_I_8"() -> (w111:dbl)
        n81 = local read "phoib_I_9"() -> (w110:dbl)
        n82 = local read "cam_avgs"() -> (w151:i32)
        n83 = case shown="\"manip\"" "scan_selector" {
          tunnel: ["delay" ("input 1") "manipulator" ("input 1") "mirror" ("input 1") "voltage" ("input 1")] -> w144
          frame "delay", Default {
          }
          frame "manip" {
          }
          frame "mirror" {
          }
          frame "volt" {
          }
        }
        n84 = local read "meas_iter"() -> (w150:i32)
        n85 = local read "ROI Right"() -> (w138:i32)
        n86 = local read "cam_exp"() -> (w143:u32)
        n87 = local read "ROI Top"() -> (w139:i32)
        n88 = local read "ESP_t0"() -> (w109:dbl)
        n89 = local read "ROI Left"() -> (w137:i32)
        n90 = local read "binning"() -> (w141:u16)
        n91 = local read "gain"() -> (w147:bool)
        n92 = Increment(x=w162) -> (x+1=w164:u16)
        n93 = Current VI's Path() -> (path=w161:path)
        n94 = call "saverunnumber.vi"("RunNumber"=w164, "VI path"=w161) -> ()  [unwired: 10 in]
        n95 = local write "RunNumber"(w164) -> ()
        n96 = Boolean To (0,1)(Boolean=w147) -> (0, 1=w142:i16)
        n97 = Boolean To (0,1)(Boolean=w146) -> (0, 1=w136:i16)
        n98 = call "create_opti_path.vi"("RunNumber"=w164, "base path"=w163) -> ("Path"=w125:path)  [unwired: 2 in]
        n99 = call "create scan vectr.vi"("Table Control"="waypoints") -> ("Array"=w119:dbl[])
        n100 = Build Path(base path=w125, name or relative path="scanvector.txt") -> (appended path=w108:path)
        n101 = Build Path(base path=w125, name or relative path="info.txt") -> (appended path=w145:path)
        n102 = Format Into String(format string="ScanType:%s\\nAverages:%u\\nRepetitions:%u\\nLensMode:%s\\nVoltageRange:%s\\nExposure:%u\\nGain:%u\\nBinning:%u\\nROIbottom:%u\\nROItop:%u\\nROIright:%u\\nROIleft:%u\\nDarkImg:%u\\nKineticEnergy:%f\\nPassEnergy:%f\\nCoilCurrent:%f\\nWorkFunction:%f\\nDetectorVoltage:%f\\nScreenVoltage:%f\\nConversionVoltage:%f\\nFocusDisplacement1:%f\\nFocusDisplacement2:%f\\nTimeZero:%f", initial string=w145, w144, w151, w150, w149, w148, w143, w142, w141, w140, w139, w138, w137, w136, w118, w117, w116, w115, w114, w113, w112, w111, w110, w109) -> ()  [unwired: 1 in, 2 out]
        n103 = Unbundle(w134) -> ("queue out"=w126:refnum<queue>, "queue out"=w133:refnum<queue>, "queue out"=w132:refnum<queue>, "queue out"=w131:refnum<queue>, "queue out"=w130:refnum<queue>)
        n104 = for {
          tunnel: w119 -> [w306] mode=indexing
          tunnel: [w305] -> w127 mode=indexing
          tunnel: [w304] -> w128
          tunnel: w133 -> [w303]
          tunnel: w132 -> [w302]
          tunnel: w131 -> [w301]
          tunnel: w130 -> [w300]
          tunnel: "scan_selector" -> [w299]
          tunnel: w108 -> [w298]
          n105 = case shown="\"mirror\"" w299 {
            tunnel: w306 -> [w314 w341 w354 w364]
            tunnel: [w312 w329 w351 w368] -> w304
            tunnel: [w318 w330 w352 w369] -> w305
            tunnel: w303 -> [w312 _ _ _]
            tunnel: w302 -> [_ w329 _ _]
            tunnel: w301 -> [_ _ _ w368]
            tunnel: w300 -> [_ _ w351 _]
            tunnel: w298 -> [w307 w324 w348 w365]
            frame "delay", Default {
              w320 = ":" ("string")
              n106 = local read "ESP_t0"() -> (w313:dbl)
              n107 = call "time2mm.vi"("fs[1]/ps[0]"=TRUE, "Offset (mm)"=w313, "time"=w314) -> ("position (mm)"=w309:dbl)
              n108 = local read "ESP Axis"() -> (w317:i32)
              n109 = Build Array(w309) -> (w308:dbl[])
              n110 = Number To Decimal String(number=w317) -> (decimal integer string=w316:string)  [unwired: 1 in]
              n111 = Number To Fractional String(number=w309) -> (F-format string=w322:string)  [unwired: 3 in]
              n112 = call-poly <vilib>:"Write Delimited Spreadsheet.vi"("file path (dialog if empty)"=w307, "format (%.3f)"="%.6f", "1D data"=w308, "append to file? (new file:F)"=TRUE ("append to file? (F)")) -> ()  [unwired: 10 in, 2 out]
              n113 = Concatenate Strings("abs:" ("string"), w316, w320, w322, w320, "wait" ("string")) -> (w318:string)
            }
            frame "manip" {
              n114 = call-poly <vilib>:"Vector Norm.vi"("Input Vector"="scan_manip_deltas") -> ("norm"=w343:dbl)  [unwired: 9 in, 1 out]
              n115 = Divide(x="scan_manip_deltas", y=w343) -> (x/y=w342:dbl[])
              n116 = Multiply(x=w342, y=w341) -> (x*y=w327:dbl[])
              n117 = Add(x="scan_manip_start", y=w327) -> (x+y=w323:dbl[])
              n118 = call-poly <vilib>:"Write Delimited Spreadsheet.vi"("file path (dialog if empty)"=w324, "format (%.3f)"="%.6f", "1D data"=w323, "append to file? (new file:F)"=TRUE ("append to file? (F)")) -> ()  [unwired: 10 in, 2 out]
              n119 = Index Array(array=w323) -> (element #1=w332:dbl, element #2=w333:dbl, element #3=w334:dbl, element #4=w335:dbl, element #5=w336:dbl, element #6=w337:dbl)  [unwired: 6 in]
              n120 = Format Into String(format string="%g_%g_%g_%g_%g_%g", w332, w333, w334, w335, w336, w337) -> (resulting string=w339:string)  [unwired: 2 in, 1 out]
              n121 = Concatenate Strings("abs:" ("string"), w339, ":wait" ("string")) -> (w330:string)
            }
            frame "mirror" {
              n122 = call-poly <vilib>:"Vector Norm.vi"("Input Vector"="scan_mirr_deltas") -> ("norm"=w362:dbl)  [unwired: 9 in, 1 out]
              n123 = Divide(x="scan_mirr_deltas", y=w362) -> (x/y=w361:dbl[])
              n124 = Multiply(x=w361, y=w354) -> (x*y=w350:dbl[])
              n125 = Add(x="scan_mirr_start", y=w350) -> (x+y=w347:dbl[])
              n126 = call-poly <vilib>:"Write Delimited Spreadsheet.vi"("file path (dialog if empty)"=w348, "format (%.3f)"="%.6f", "1D data"=w347, "append to file? (new file:F)"=TRUE ("append to file? (F)")) -> ()  [unwired: 10 in, 2 out]
              n127 = Index Array(array=w347) -> (element #1=w357:dbl, element #2=w358:dbl)  [unwired: 2 in]
              n128 = Format Into String(format string="%g_%g", w357, w358) -> (resulting string=w360:string)  [unwired: 2 in, 1 out]
              n129 = Concatenate Strings("abs:" ("string"), w360, ":wait" ("string")) -> (w352:string)
            }
            frame "volt" {
              n130 = local read "scan_volt_parameter"() -> (w372:string)
              n131 = Build Array(w364) -> (w363:dbl[])
              n132 = Number To Fractional String(number=w364) -> (F-format string=w370:string)  [unwired: 3 in]
              n133 = Concatenate Strings("setsgl:" ("string"), w372, ":" ("string"), w370) -> (w369:string)
              n134 = call-poly <vilib>:"Write Delimited Spreadsheet.vi"("file path (dialog if empty)"=w365, "format (%.3f)"="%.6f", "1D data"=w363, "append to file? (new file:F)"=TRUE ("append to file? (F)")) -> ()  [unwired: 10 in, 2 out]
            }
          }
        }
        n135 = Build Path(base path=w125, name or relative path="RAW\\LUT.txt") -> (appended path=w123:path)
        n136 = call-poly <vilib>:"Write Delimited Spreadsheet.vi"("file path (dialog if empty)"=w123, "1D data"=string[] ["filename", "time", "delaystage", "X", "Y", "Z", "polar", "tilt", "azimuth", "mirrorX", "mirrorY", "KineticEnergy", "PassEnergy", "CoilCurrent", "WorkFunction", "DetectorVoltage", "ScreenVoltage", "ConversionVoltage", "FD1", "FD2"]) -> ("new file path (Not A Path if cancelled)"=w122:path)  [unwired: 12 in, 1 out]
        n137 = Get Date/Time In Seconds() -> (seconds since 1Jan1904=w135:timestamp)
        n138 = while {
          tunnel: w125 -> [w183]
          tunnel: w158 -> [w182]
          shift-right: [w181] -> w156
          shift-left: dbl[][][] [] -> [w180]
          tunnel: w155 -> [w179]
          tunnel: w135 -> [w178]
          tunnel: w128 -> [w177]
          tunnel: w127 -> [w176]
          tunnel: w126 -> [w175]
          shift-right: [w173] -> _
          shift-left: w122 -> [w174]
          shift-right: [w172] -> w120
          shift-left: w119 -> [w171]
          i -> [w170]
          stop <- w167 stop-if-true
          n139 = local read "meas_iter"() -> (w169:i32)
          n140 = for {
            N -> [w211]
            tunnel: w183 -> [w208]
            tunnel: w182 -> [w233]
            tunnel: w170 -> [w206]
            shift-right: [w222] -> w181
            shift-left: w180 -> [w229]
            tunnel: w179 -> [w224]
            tunnel: w178 -> [w210]
            tunnel: w177 -> [w202]
            tunnel: w176 -> [w201] mode=indexing
            tunnel: w175 -> [w200]
            shift-right: [w196] -> w173
            shift-left: w174 -> [w197]
            shift-right: [w192] -> w172
            shift-left: w171 -> [w192]
            tunnel: [w189] -> w166
            tunnel: w169 -> [w188]
            i -> [w207]
            stop <- "stop after step" stop-if-true
            n141 = Cancel Notification(0:w224) -> (11:w225:errorcluster)  [unwired: 1 in, 2 out]
            n142 = Enqueue Element(queue=w202, element=w201, error in (no error)=w225) -> (error out=w228:errorcluster)  [unwired: 1 in, 2 out]
            n143 = Equal To 0?(x=w207) -> (x = 0?=w232:bool)
            n144 = Equal To 0?(x=w206) -> (x = 0?=w231:bool)
            n145 = Get Date/Time In Seconds() -> (seconds since 1Jan1904=w198:timestamp)
            n146 = Wait on Notification(notifier=w224, error in (no error)=w228) -> (error out=w227:errorcluster)  [unwired: 2 in, 3 out]
            n147 = And(x=w232, y=w231) -> (x .and. y?=w230:bool)
            n148 = Enqueue Element(queue=w200, element="snap", error in (no error)=w227) -> (error out=w226:errorcluster)  [unwired: 1 in, 2 out]
            n149 = call "createFileStruc.vi"("i_iter"=w206, "i_delay"=w207, "meas_path"=w208) -> ("AVG file"=w203:path, "RAW file"=w194:path)  [unwired: 7 in]
            n150 = Dequeue Element(queue=w233, error in (no error)=w226) -> (element=w205:dbl[][], error out=w195:errorcluster)  [unwired: 1 in, 2 out]
            n151 = Strip Path(path=w194) -> (name=w193:string)  [unwired: 1 out]
            n152 = Array Size(array=w205) -> (size(s)=w237:i32[])
            n153 = call-poly <vilib>:"Write Delimited Spreadsheet.vi"("file path (dialog if empty)"=w194, "2D data"=w205, "error in (no error)"=w195) -> ()  [unwired: 11 in, 2 out]
            n154 = Index Array(array=w237) -> (element #1=w235:i32, element #2=w234:i32)  [unwired: 2 in]
            n155 = Subtract(x=w198, y=w210) -> (x-y=w214:dbl)
            n156 = flat-sequence {
              tunnel: "%s\\t%<%Y.%m.%d %H:%M:%S>T\\t%f\\t%f\\t%f\\t%f\\t%f\\t%f\\t%f\\t%f\\t%f\\t%f\\t%f\\t%f\\t%f\\t%f\\t%f\\t%f\\t%f\\t%f\\t%f" -> [w267]
              tunnel: w198 -> [w266]
              tunnel: w197 -> [w243]
              tunnel: [w242] -> w196
              tunnel: w195 -> [w239]
              tunnel: w193 -> [w238]
              frame #0 {
                n157 = local read "pos"() -> (w268:dbl[])
                n158 = local read "mirr_posX"() -> (w255:i32)
                n159 = local read "mirr_posY"() -> (w256:i32)
                n160 = local read "ESP_delay"() -> (w248:dbl)
                n161 = local read "phoib_I_1"() -> (w257:dbl)
                n162 = local read "phoib_I_2"() -> (w258:dbl)
                n163 = local read "phoib_I_3"() -> (w259:dbl)
                n164 = local read "phoib_I_4"() -> (w260:dbl)
                n165 = local read "phoib_I_5"() -> (w261:dbl)
                n166 = local read "phoib_I_6"() -> (w262:dbl)
                n167 = local read "phoib_I_7"() -> (w263:dbl)
                n168 = local read "phoib_I_8"() -> (w264:dbl)
                n169 = local read "phoib_I_9"() -> (w265:dbl)
                n170 = local read "ESP_pos"() -> (w247:dbl)
                n171 = Index Array(array=w268) -> (element #1=w249:dbl, element #2=w250:dbl, element #3=w251:dbl, element #4=w252:dbl, element #5=w253:dbl, element #6=w254:dbl)  [unwired: 6 in]
                n172 = Format Into String(format string=w267, error in=w239, w238, w266, w247, w248, w249, w250, w251, w252, w253, w254, w255, w256, w257, w258, w259, w260, w261, w262, w263, w264, w265) -> (resulting string=w245:string)  [unwired: 1 in, 1 out]
                n173 = Spreadsheet String To Array(format string="%s", spreadsheet string=w245, array type (2D Dbl)=string[] []) -> (array=w241:string[])  [unwired: 1 in]
                n174 = call-poly <vilib>:"Write Delimited Spreadsheet.vi"("file path (dialog if empty)"=w243, "1D data"=w241, "append to file? (new file:F)"=TRUE ("append to file? (F)")) -> ("new file path (Not A Path if cancelled)"=w242:path)  [unwired: 11 in, 1 out]
              }
            }
            n175 = case shown="True" w230 {
              tunnel: w211 -> [_ w274]
              tunnel: [w269 w272] -> w236
              tunnel: w229 -> [w269 _]
              tunnel: w235 -> [_ w271]
              tunnel: w234 -> [_ w270]
              frame False {
              }
              frame True {
                n176 = Initialize Array(0.0 ("element"), w274, w271, w270) -> (w272:dbl[][][])
              }
            }
            n177 = Increment(x=w207) -> (x+1=w218:i32)
            "current scan" <- w218
            n178 = Increment(x=w206) -> (x+1=w217:i32)
            "current iteration" <- w217
            n179 = for {
              N: w235 -> [_]
              tunnel: w207 -> [w281]
              shift-right: [w279] -> w222
              shift-left: w236 -> [w282]
              tunnel: w206 -> [w277]
              shift-right: [w276] -> w204
              shift-left: w205 -> [w278]
              tunnel: w234 -> [w275]
              i -> [w280]
              n180 = for {
                N: w275 -> [_]
                tunnel: w281 -> [w289]
                tunnel: w280 -> [w286]
                shift-right: [w288] -> w279
                shift-left: w282 -> [w290]
                tunnel: w277 -> [w284]
                shift-right: [w283] -> w276
                shift-left: w278 -> [w287]
                i -> [w285]
                n181 = in-place {
                  in-place-border: w284 -> [w296]
                  n182 = in-place-array #1(w290, w289, w286, w285) -> (w297:dbl)
                  n183 = in-place-array #2(w287, w286, w285) -> (w294:dbl)
                  n184 = Multiply(x=w297, y=w296) -> (x*y=w295:dbl)
                  n185 = Increment(x=w296) -> (x+1=w292:i32)
                  n186 = Add(x=w295, y=w294) -> (x+y=w293:dbl)
                  n187 = Divide(x=w293, y=w292) -> (x/y=w291:dbl)
                  n188 = in-place-array #1(w291) -> (w288:dbl[][][])  [unwired: 3 out]
                  n189 = in-place-array #2(w291) -> (w283:dbl[][])  [unwired: 2 out]
                }
              }
            }
            n190 = Multiply(x=w211, y=w206) -> (x*y=w213:i32)
            n191 = Multiply(x=w211, y=w188) -> (x*y=w209:i32)
            n192 = Divide(x=w218, y=w211) -> (x/y=→"scan":dbl)
            n193 = Divide(x=w217, y=w188) -> (x/y=→"iteration":dbl)
            n194 = Add(x=w207, y=w213) -> (x+y=w212:i32)
            n195 = Divide(x=w214, y=w212) -> (x/y=w184:dbl)
            n196 = Multiply(x=w184, y=w209) -> (x*y=w187:dbl)
            n197 = local write "time/step [s]"(w184) -> ()
            n198 = local write "duration [HH:MM:SS]"(w187) -> ()
            n199 = property on="mainimg" class="IntGraph (strict)"() -> ("CrsrLis"=w221:T4)  [unwired: 2 in, 2 out]
            n200 = call-poly <vilib>:"Write Delimited Spreadsheet.vi"("file path (dialog if empty)"=w203, "2D data"=w204) -> ()  [unwired: 12 in, 2 out]
            n201 = call "processData.vi"("Cursor List"=w221, "data in"=w222) -> ("Angle Chart"=→"anglegraph":dbl[][], "Energy Chart"=→"energygraph":dbl[][], "Intensity Chart"=w220:dbl[])  [unwired: 1 in]
            n202 = Bundle("Array"=w192, "Intensity Chart"=w220) -> (→"intensitygraph":cluster{"Array":dbl[], "Intensity Chart":dbl[]})  [unwired: 1 in]
            n203 = Or(x="stop after iteration", y="stop after step") -> (x .or. y?=w189:bool)
          }
          n204 = Increment(x=w170) -> (x+1=w168:i32)
          n205 = Greater Or Equal?(x=w168, y=w169) -> (x >= y?=w165:bool)
          n206 = Or(x=w166, y=w165) -> (x .or. y?=w167:bool)
        }
      }
      frame "refresh" {
        n207 = Dequeue Element(queue=w378) -> ()  [unwired: 2 in, 4 out]
        n208 = property on="mainimg" class="IntGraph (strict)"() -> ("CrsrLis"=w385:T4)  [unwired: 2 in, 2 out]
        n209 = call "processData.vi"("Cursor List"=w385, "data in"=w384) -> ("Angle Chart"=w382:dbl[][], "Energy Chart"=w383:dbl[][], "Intensity Chart"=w379:dbl[])  [unwired: 1 in]
        n210 = Bundle("Array"=w380, "Intensity Chart"=w379) -> (w381:cluster{"Array":dbl[], "Intensity Chart":dbl[]})  [unwired: 1 in]
        n211 = local write "energygraph"(w383) -> ()
        n212 = local write "intensitygraph"(w381) -> ()
        n213 = local write "anglegraph"(w382) -> ()
      }
    }
  }
  n214 = while {
    tunnel: w14 -> [w393]
    tunnel: w13 -> [w392]
    tunnel: w12 -> [w391]
    tunnel: w11 -> [w390]
    tunnel: w16 -> [w388]
    tunnel: w23 -> [w389]
    tunnel: w3 -> [w387]
    tunnel: w4 -> [w386]
    stop <- w394 stop-if-true
    n215 = event shown="[12] \"meas_iter\", \"waypoints\": Value Change" {
      selector: _ -> [_ _ _ _ _ _ _ _ _ _ _ _ _ _ _ _ _ _ _ _ _ _ _ _ _ _ _ _ _]
      dyn-events: _ -> [_ _ _ _ _ _ _ _ _ _ _ _ _ _ _ _ _ _ _ _ _ _ _ _ _ _ _ _ _]
      timeout: _ -> [_ _ _ _ _ _ _ _ _ _ _ _ _ _ _ _ _ _ _ _ _ _ _ _ _ _ _ _ _]
      tunnel: [_ TRUE _ _ _ _ _ _ _ _ _ _ _ _ _ _ _ _ _ _ _ _ _ _ _ _ _ _ _] -> w394
      tunnel: w393 -> [_ w406 w419 _ _ _ _ _ w445 w447 _ _ _ _ _ _ _ _ _ _ _ _ _ _ _ _ _ _ _]
      tunnel: w392 -> [_ w405 _ w423 _ _ _ _ _ _ _ _ _ _ _ _ _ _ _ w512 _ _ w534 _ _ _ _ _ _]
      tunnel: w391 -> [_ w404 _ _ w429 _ _ _ _ _ _ _ _ _ _ _ w487 w502 w504 _ _ _ _ _ _ _ _ _ _]
      tunnel: w390 -> [_ w403 _ _ _ w435 w441 w442 _ _ _ _ _ _ _ _ _ _ _ _ _ _ _ _ _ _ _ _ _]
      tunnel: w389 -> [_ w412 _ _ _ _ _ _ _ _ _ _ _ _ _ _ _ _ _ _ _ _ _ _ _ _ _ _ _]
      tunnel: w388 -> [_ w402 _ _ _ _ _ _ _ _ w449 w451 _ _ _ _ _ _ _ _ _ _ _ _ _ _ w553 _ _]
      tunnel: w387 -> [_ w411 _ _ _ _ _ _ _ _ _ _ _ _ _ _ _ _ _ _ _ _ _ _ _ _ _ _ _]
      tunnel: w386 -> [_ w401 _ _ _ _ _ _ _ _ _ _ _ w465 _ _ _ _ _ _ _ _ _ _ _ _ _ w555 w576]
      event Timeout {
        n216 = event-data() -> ()  [unwired: 1 in, 1 out]
      }
      event "main_close": Value Change {
        w407 = "close" ("element")
        w408 = "release" ("element")
        n217 = event-data() -> ()  [unwired: 1 in, 1 out]
        n218 = Flush Queue(queue=w406) -> (queue out=w400:refnum<queue>)  [unwired: 1 in, 2 out]
        n219 = Flush Queue(queue=w405) -> (queue out=w399:refnum<queue>)  [unwired: 1 in, 2 out]
        n220 = Flush Queue(queue=w404) -> (queue out=w398:refnum<queue>)  [unwired: 1 in, 2 out]
        n221 = Flush Queue(queue=w403) -> (queue out=w397:refnum<queue>)  [unwired: 1 in, 2 out]
        n222 = Flush Queue(queue=w402) -> (queue out=w396:refnum<queue>)  [unwired: 1 in, 2 out]
        n223 = Flush Queue(queue=w401) -> (queue out=w395:refnum<queue>)  [unwired: 1 in, 2 out]
        n224 = Release Notifier(notifier=w411) -> ()  [unwired: 2 in, 3 out]
        n225 = Release Queue(queue=w412) -> ()  [unwired: 2 in, 3 out]
        n226 = Enqueue Element(queue=w400, element=w408) -> (queue out=w416:refnum<queue>)  [unwired: 2 in, 2 out]
        n227 = Enqueue Element(queue=w399, element=w408) -> (queue out=w415:refnum<queue>)  [unwired: 2 in, 2 out]
        n228 = Enqueue Element(queue=w398, element=w408) -> (queue out=w414:refnum<queue>)  [unwired: 2 in, 2 out]
        n229 = Enqueue Element(queue=w397, element=w408) -> (queue out=w413:refnum<queue>)  [unwired: 2 in, 2 out]
        n230 = Enqueue Element(queue=w395, element=w408) -> (queue out=w410:refnum<queue>, error out=w409:errorcluster)  [unwired: 2 in, 1 out]
        n231 = Enqueue Element(queue=w416, element=w407) -> ()  [unwired: 2 in, 3 out]
        n232 = Enqueue Element(queue=w415, element=w407) -> ()  [unwired: 2 in, 3 out]
        n233 = Enqueue Element(queue=w414, element=w407) -> ()  [unwired: 2 in, 3 out]
        n234 = Enqueue Element(queue=w413, element=w407) -> ()  [unwired: 2 in, 3 out]
        n235 = Enqueue Element(queue=w396, element=w407) -> ()  [unwired: 2 in, 3 out]
        n236 = Enqueue Element(queue=w410, element=w407, error in (no error)=w409) -> ()  [unwired: 1 in, 3 out]
      }
      event "cam_release", "cam_init": Value Change {
        n237 = event-data() -> ()  [unwired: 1 in, 2 out]
        n238 = Select(t="init" ("name (unnamed)"), s="cam_init", f="release" ("name (unnamed)")) -> (s? t:f=w418:string)
        n239 = Enqueue Element(queue=w419, element=w418) -> ()  [unwired: 2 in, 3 out]
      }
      event "ESP_release", "ESP_init": Value Change {
        n240 = event-data() -> ()  [unwired: 1 in, 2 out]
        n241 = Select(t="init" ("name (unnamed)"), s="ESP_init", f="release" ("name (unnamed)")) -> (s? t:f=w427:string)
        n242 = Enqueue Element(queue=w423, element=w427) -> ()  [unwired: 2 in, 3 out]
      }
      event "manip_init", "manip_release": Value Change {
        n243 = event-data() -> ()  [unwired: 1 in, 2 out]
        n244 = Flush Queue(queue=w429) -> (queue out=w428:refnum<queue>)  [unwired: 1 in, 2 out]
        n245 = Select(t="init" ("name (unnamed)"), s="manip_init", f="release" ("name (unnamed)")) -> (s? t:f=w431:string)
        n246 = Enqueue Element(queue=w428, element=w431) -> ()  [unwired: 2 in, 3 out]
      }
      event "phoib_release", "phoib_init": Value Change {
        n247 = event-data() -> ()  [unwired: 1 in, 2 out]
        n248 = Flush Queue(queue=w435) -> (queue out=w434:refnum<queue>)  [unwired: 1 in, 2 out]
        n249 = Select(t="init" ("name (unnamed)"), s="phoib_init", f="release" ("name (unnamed)")) -> (s? t:f=w437:string)
        n250 = Enqueue Element(queue=w434, element=w437) -> ()  [unwired: 2 in, 3 out]
      }
      event "phoib_standby": Value Change {
        n251 = event-data() -> ()  [unwired: 1 in, 2 out]
        n252 = Enqueue Element(queue=w441, element="standby") -> ()  [unwired: 2 in, 3 out]
      }
      event "phoib_set": Value Change {
        n253 = event-data() -> ()  [unwired: 1 in, 2 out]
        n254 = Enqueue Element(queue=w442, element="set") -> ()  [unwired: 2 in, 3 out]
      }
      event "cam_dark": Value Change {
        n255 = event-data() -> ()  [unwired: 1 in, 2 out]
        n256 = Enqueue Element(queue=w445, element="dark") -> ()  [unwired: 2 in, 3 out]
      }
      event "ROI Left", "ROI Right", "ROI Top", "ROI Bottom", "cam_exp", "binning", "gain": Value Change {
        n257 = event-data() -> ()  [unwired: 1 in, 1 out]
        n258 = Enqueue Element(queue=w447, element="set") -> ()  [unwired: 2 in, 3 out]
      }
      event "cam_saveimg": Value Change {
        n259 = event-data() -> ()  [unwired: 1 in, 1 out]
        n260 = Enqueue Element(queue=w449, element="single") -> ()  [unwired: 2 in, 3 out]
      }
      event "scan_go": Value Change {
        n261 = event-data() -> ()  [unwired: 1 in, 1 out]
        n262 = Enqueue Element(queue=w451, element="scan") -> ()  [unwired: 2 in, 3 out]
      }
      event "meas_iter", "waypoints": Value Change {
        n263 = event-data() -> ()  [unwired: 1 in, 6 out]
        n264 = local read "waypoints"() -> (w463:string[][])
        n265 = local read "meas_iter"() -> (w457:i32)
        n266 = local read "binning"() -> (w460:u16)
        n267 = call "create scan vectr.vi"("Table Control"=w463) -> ("Array"=w462:dbl[])
        n268 = Index Array(array=dbl[] [8.79, 2.2, 0.553, 0.138], index=w460) -> (element=w456:dbl)
        n269 = Array Size(array=w462) -> (size(s)=w459:i32)
        "measpoints" <- w459
        n270 = Multiply(x=w459, y=w457) -> (x*y=w454:i32)
        "total steps" <- w454
        n271 = Multiply(x=w454, y="time/step [s]") -> (x*y=→"duration [HH:MM:SS]":dbl)
        n272 = Multiply(x=w459, y=w456) -> (x*y=→"RAM [MB]":dbl)
        n273 = Multiply(x=w454, y=w456) -> (x*y=→"disk [MB]":dbl)
      }
      event "mirr_go": Value Change {
        n274 = event-data() -> ()  [unwired: 1 in, 1 out]
        n275 = Index Array(array="mirr_dest") -> (element #1=w470:i32, element #2=w469:i32)  [unwired: 2 in]
        n276 = Format Into String(format string="%g_%g", w470, w469) -> (resulting string=w467:string)  [unwired: 2 in, 1 out]
        n277 = Concatenate Strings("abs:" ("string"), w467) -> (w464:string)
        n278 = Enqueue Element(queue=w465, element=w464) -> ()  [unwired: 2 in, 3 out]
      }
      event "scan_manip_setstart": Value Change {
        n279 = event-data() -> ()  [unwired: 1 in, 1 out]
        n280 = local read "pos"() -> (w472:dbl[])
        n281 = local write "scan_manip_start"(w472) -> ()
      }
      event "scan_mirr_setstart": Value Change {
        n282 = event-data() -> ()  [unwired: 1 in, 1 out]
        n283 = local read "mirr_posX"() -> (w475:i32)
        n284 = local read "mirr_posY"() -> (w474:i32)
        n285 = Build Array(w475, w474) -> (w473:i32[])
        n286 = local write "scan_mirr_start"(w473) -> ()
      }
      event "Move Abs": Value Change {
        n287 = event-data() -> ()  [unwired: 1 in, 1 out]
        n288 = Index Array(array="dest") -> (element #1=w485:dbl, element #2=w484:dbl, element #3=w483:dbl, element #4=w482:dbl, element #5=w481:dbl, element #6=w480:dbl)  [unwired: 6 in]
        n289 = Format Into String(format string="%g_%g_%g_%g_%g_%g", w485, w484, w483, w482, w481, w480) -> (resulting string=w478:string)  [unwired: 2 in, 1 out]
        n290 = Concatenate Strings("abs:" ("string"), w478) -> (w477:string)
        n291 = Enqueue Element(queue=w487, element=w477) -> ()  [unwired: 2 in, 3 out]
      }
      event "ManipRel +", "ManipRel -": Value Change {
        n292 = event-data() -> ()  [unwired: 1 in, 2 out]
        n293 = Negate(x="manip_deltas") -> (-x=w490:dbl[])
        n294 = Select(t="manip_deltas", s="ManipRel +", f=w490) -> (s? t:f=w488:dbl[])
        n295 = Index Array(array=w488) -> (element #1=w494:dbl, element #2=w495:dbl, element #3=w496:dbl, element #4=w497:dbl, element #5=w498:dbl, element #6=w499:dbl)  [unwired: 6 in]
        n296 = Format Into String(format string="%g_%g_%g_%g_%g_%g", w494, w495, w496, w497, w498, w499) -> (resulting string=w501:string)  [unwired: 2 in, 1 out]
        n297 = Concatenate Strings("rel:" ("string"), w501) -> (w492:string)
        n298 = Enqueue Element(queue=w502, element=w492) -> ()  [unwired: 2 in, 3 out]
      }
      event "stop manip": Value Change {
        n299 = event-data() -> ()  [unwired: 1 in, 1 out]
        n300 = Enqueue Element(queue=w504, element="stop") -> ()  [unwired: 2 in, 3 out]
      }
      event "ESP_go": Value Change {
        w506 = ":" ("string")
        n301 = event-data() -> ()  [unwired: 1 in, 1 out]
        n302 = local read "ESP Axis"() -> (w505:i32)
        n303 = Number To Decimal String(number=w505) -> (decimal integer string=w508:string)  [unwired: 1 in]
        n304 = Number To Fractional String(number="ESP_dest") -> (F-format string=w507:string)  [unwired: 3 in]
        n305 = Concatenate Strings("abs:" ("string"), w508, w506, w507, w506) -> (w511:string)
        n306 = Enqueue Element(queue=w512, element=w511) -> ()  [unwired: 2 in, 3 out]
      }
      event "ESP_set_t0": Value Change {
        n307 = event-data() -> ()  [unwired: 1 in, 1 out]
        n308 = Current VI's Path() -> (path=w523:path)
        n309 = Strip Path(path=w523) -> (stripped path=w521:path)  [unwired: 1 out]
        n310 = Strip Path(path=w521) -> (stripped path=w520:path)  [unwired: 1 out]
        n311 = local read "ESP_pos"() -> (w522:dbl)
        "ESP_t0" <- w522
        n312 = Number To Fractional String(number=w522) -> (F-format string=w515:string)  [unwired: 3 in]
        n313 = Build Path(base path=w520, name or relative path="t0.txt") -> (appended path=w517:path)
        n314 = Get Date/Time In Seconds() -> (seconds since 1Jan1904=w519:timestamp)
        n315 = Format Date/Time String(time format string (%c)="%Y.%m.%d %H:%M", seconds (now)=w519) -> (date/time string=w516:string)  [unwired: 1 in]
        n316 = Build Array(w516, w515) -> (w514:string[])
        n317 = call-poly <vilib>:"Write Delimited Spreadsheet.vi"("file path (dialog if empty)"=w517, "1D data"=w514, "append to file? (new file:F)"=TRUE ("append to file? (F)")) -> ()  [unwired: 11 in, 2 out]
      }
      event "ESP_opent0file": Value Change {
        n318 = event-data() -> ()  [unwired: 1 in, 6 out]
        n319 = Current VI's Path() -> (path=w527:path)
        n320 = Strip Path(path=w527) -> (stripped path=w526:path)  [unwired: 1 out]
        n321 = Strip Path(path=w526) -> (stripped path=w528:path)  [unwired: 1 out]
        n322 = call <vilib>:"System Exec.vi"("wait until completion? (T)"=FALSE, "working directory"=w528, "command line"="notepad t0.txt") -> ()  [unwired: 5 in, 4 out]
      }
      event "ESP_+", "ESP_-": Value Change {
        n323 = event-data() -> ()  [unwired: 1 in, 6 out]
        n324 = local read "ESP Axis"() -> (w530:i32)
        n325 = Negate(x="ESP_delta") -> (-x=w537:dbl)
        n326 = Select(t="ESP_delta", s="ESP_+", f=w537) -> (s? t:f=w535:dbl)
        n327 = Number To Decimal String(number=w530) -> (decimal integer string=w533:string)  [unwired: 1 in]
        n328 = Number To Fractional String(number=w535) -> (F-format string=w531:string)  [unwired: 3 in]
        n329 = Concatenate Strings("rel:" ("string"), w533, ":" ("string"), w531) -> (w540:string)
        n330 = Enqueue Element(queue=w534, element=w540) -> ()  [unwired: 2 in, 3 out]
      }
      event "ESP_dest": Value Change {
        n331 = event-data() -> ()  [unwired: 1 in, 6 out]
        n332 = local read "ESP_dest"() -> (w544:dbl)
        n333 = local read "ESP_t0"() -> (w543:dbl)
        n334 = call "mm2time.vi"("fs?"=TRUE ("fs[1]/ps[0]"), "Offset (mm)"=w543, "distance (mm)"=w544) -> ("time in fs/ps seconds"=w541:dbl)
        n335 = local write "ESP_dest_t"(w541) -> ()
      }
      event "ESP_dest_t": Value Change {
        n336 = event-data() -> ()  [unwired: 1 in, 1 out]
        n337 = local read "ESP_t0"() -> (w547:dbl)
        n338 = call "time2mm.vi"("fs[1]/ps[0]"=TRUE, "Offset (mm)"=w547, "time"="ESP_dest_t") -> ("position (mm)"=w545:dbl)
        n339 = local write "ESP_dest"(w545) -> ()
      }
      event "load delay table": Value Change {
        n340 = event-data() -> ()  [unwired: 1 in, 6 out]
        n341 = call-poly <vilib>:"Read Delimited Spreadsheet.vi"() -> ("all rows"=w550:string[][], "error out"=w549:errorcluster)  [unwired: 10 in, 4 out]
        n342 = case shown="No Error" w549 {
          tunnel: w550 -> [w551 _]
          frame No Error {
            n343 = local write "waypoints"(w551) -> ()
          }
          frame Error {
          }
        }
      }
      event "mainimg": Cursor Release {
        n344 = event-data() -> ()  [unwired: 1 in, 1 out]
        n345 = Enqueue Element(queue=w553, element="refresh") -> ()  [unwired: 2 in, 3 out]
      }
      event "mirr_init", "mirr_release": Value Change {
        n346 = event-data() -> ()  [unwired: 1 in, 6 out]
        n347 = Flush Queue(queue=w555) -> (queue out=w556:refnum<queue>)  [unwired: 1 in, 2 out]
        n348 = Select(t="init" ("name (unnamed)"), s="mirr_init", f="release" ("name (unnamed)")) -> (s? t:f=w557:string)
        n349 = Enqueue Element(queue=w556, element=w557) -> ()  [unwired: 2 in, 3 out]
      }
      event "mirr_X-", "mirr_X+", "mirr_Y+", "mirr_Y-": Value Change {
        n350 = event-data() -> ()  [unwired: 1 in, 1 out]
        n351 = local read "mirr_X#"() -> (w567:u8)
        n352 = local read "mirr_Y#"() -> (w566:u8)
        n353 = Or(x="mirr_X+", y="mirr_X-") -> (x .or. y?=w568:bool)
        n354 = Or(x="mirr_X-", y="mirr_Y-") -> (x .or. y?=w574:bool)
        n355 = Negate(x="mirr_rel") -> (-x=w573:i32)
        n356 = Select(t=w567, s=w568, f=w566) -> (s? t:f=w565:u8)
        n357 = Select(t=w573, s=w574, f="mirr_rel") -> (s? t:f=w562:i32)
        n358 = Number To Decimal String(number=w565) -> (decimal integer string=w564:string)  [unwired: 1 in]
        n359 = Number To Decimal String(number=w562) -> (decimal integer string=w561:string)  [unwired: 1 in]
        n360 = Concatenate Strings("rel:" ("string"), w564, ":" ("string"), w561) -> (w560:string)
        n361 = Enqueue Element(queue=w576, element=w560) -> ()  [unwired: 2 in, 3 out]
      }
    }
  }
  n362 = while {
    tunnel: w14 -> [w603]
    shift-right: [w597] -> _
    shift-left: _ -> [w596]
    shift-right: [w595] -> _
    shift-left: _ -> [w593]
    shift-right: [w594] -> _
    shift-left: _ -> [w592]
    shift-right: [w589] -> _
    shift-left: 0 -> [w590]
    shift-right: [w588] -> _
    shift-left: _ -> [w587]
    shift-right: [w586] -> _
    shift-left: _ -> [w585]
    tunnel: w23 -> [w584]
    shift-right: [w583] -> _
    shift-left: _ -> [w582]
    shift-right: [w580] -> _
    shift-left: _ -> [w579]
    shift-right: [w578] -> _
    shift-left: _ -> [w577]
    i -> [w581]
    stop <- w591 stop-if-true
    # "cam"
    n363 = Preview Queue Element(queue=w603, timeout in ms (-1)=w590) -> (queue out=w602:refnum<queue>, element=w601:string)  [unwired: 1 in, 2 out]
    n364 = Match Pattern(string=w601, regular expression=":") -> (before substring=w598:string, after substring=w599:string)  [unwired: 1 in, 2 out]
    n365 = case shown="\"idle\", Default" w598 {
      tunnel: w602 -> [w615 w647 w680 w693 _ w781 w811 w876]
      tunnel: w599 -> [_ _ _ _ _ _ _ _]
      tunnel: [w609 w634 w679 w691 w734 w778 w796 w874] -> w597
      tunnel: w596 -> [_ _ w679 w691 w734 w778 w796 w874]
      tunnel: [w614 w648 u64 0 ("Hout") w690 w738 w779 w806 w873] -> w595
      tunnel: [w616 w649 w676 w689 w739 w780 w797 w872] -> w594
      tunnel: w593 -> [_ w651 w678 w690 w741 w783 w808 w873]
      tunnel: w592 -> [_ w650 _ w689 w740 w782 w807 w872]
      tunnel: [_ _ _ TRUE _ _ _ _] -> w591
      tunnel: [_ _ -1 _ _ _ _ -1] -> w589
      tunnel: [w608 w635 _ _ w748 _ _ _] -> w588
      tunnel: w587 -> [w608 w635 _ _ w747 _ _ _]
      tunnel: [w609 w637 w674 w688 w743 w772 w809 w871] -> w586
      tunnel: w585 -> [_ w637 w674 w688 w743 _ w809 w871]
      tunnel: w584 -> [_ _ _ _ _ _ w800 _]
      tunnel: [w606 w632 w673 w686 w701 w769 w803 w870] -> w583
      tunnel: w582 -> [w606 w632 w673 w686 w736 w769 w803 w870]
      tunnel: w581 -> [_ _ _ _ w709 _ _ _]
      tunnel: [w607 w633 w672 w687 w735 w768 w802 w869] -> w580
      tunnel: w579 -> [w607 w633 w672 w687 w708 w768 w802 w869]
      tunnel: [w605 w629 refnum<k21> refnum ("task out") w685 w694 w767 w793 w868] -> w578
      tunnel: w577 -> [_ w629 w671 w685 w694 w767 w794 w868]
      frame "init" {
        w609 = u16[][] []
        n366 = flat-sequence {
          tunnel: [w618] -> w613
          tunnel: [w619] -> w612
          tunnel: [w627] -> w614
          tunnel: [w628] -> w616
          tunnel: w613 -> [w628]
          tunnel: w612 -> [w627]
          frame #0 {
            n367 = local write "cam_con?"(FALSE ("cam_con?")) -> ()
          }
          frame #1 {
            n368 = call "SCInitBoard.vi"("boardnr"="board number") -> ("Hout"=w622:u32, "error out"=w623:errorcluster)  [unwired: 1 in, 1 out]
            n369 = call "SCSetupCamera.vi"("Handle"=w622, "error in (no error)"=w623) -> ("Hout"=w624:u64, "error out"=w625:errorcluster)  [unwired: 1 out]
            n370 = call "SCStopCOC.vi"("error in (no error)"=w625, "Stop mode"=0, "Handle"=w624) -> ("error out"=w618:errorcluster, "Hout"=w619:u64)
          }
          frame #2 {
            n371 = local write "cam_con?"(TRUE ("cam_con?")) -> ()
          }
        }
        n372 = Dequeue Element(queue=w615) -> (queue out=w611:refnum<queue>)  [unwired: 2 in, 3 out]
        n373 = Enqueue Element At Opposite End(queue=w611, element="set") -> ()  [unwired: 2 in, 3 out]
        n374 = call-poly <vilib>:"DAQmx Create Virtual Channel.vi"("lines"=tag "Dev2/port0/line7") -> ("task out"=w605:refnum<k21>)  [unwired: 13 in, 1 out]
      }
      frame "set" {
        n375 = Dequeue Element(queue=w647) -> ()  [unwired: 2 in, 4 out]
        n376 = call "SCStopCOC.vi"("error in (no error)"=w650, "Stop mode"=0, "Handle"=w651) -> ("error out"=w666:errorcluster, "Hout"=w665:u64)
        n377 = Bundle By Name(cluster=cluster{"Delay":dbl, "Exposure ":dbl} {"Delay"=0.0, "Exposure "=0.0} ("Delay and exposure"), "Exposure"="cam_exp") -> (w644:cluster{"Delay":dbl, "Exposure ":dbl})
        n378 = Bundle By Name(cluster=T5 {"Camera type"=0, "Operating mode\nHP & QE / HS & DiCam Pro "=0, "Frame trigger \n(High Performance and QE only)"=0, "Sequence trigger"=0, "Low Light\n(QE only)"=FALSE, "Gain"=FALSE, "Horzontal\nbinning"=0, "Vertical\nbinning "=0, "ROI Left"=1, "ROI Right"=20, "ROI Top"=1, "ROI Bottom"=15} ("Camera controls"), "Operating mode\nHP & QE / HS & DiCam Pro"="Operating mode\nHP & QE / HS & DiCam Pro", "Horzontal\nbinning"="binning", "Vertical\nbinning"="binning", "ROI Left"="ROI Left", "ROI Right"="ROI Right", "ROI Top"="ROI Top", "ROI Bottom"="ROI Bottom", "Gain"="gain", "Frame trigger \n(High Performance and QE only)"="Frame trigger \n(High Performance and QE only)") -> (w661:T5)
        n379 = call "New delay and exposure forma.vi"("Operating mode\nHP & QE / HS & DiCam Pro"="Operating mode\nHP & QE / HS & DiCam Pro", "Delay and exposure"=w644) -> ("Output table"=w662:string)  [unwired: 3 in]
        n380 = call "SCSetCoC.vi"("error in (no error)"=w666, "Delay and exposure table"=w662, "Camera controls"=w661, "Handle"=w665) -> ("error out"=w654:errorcluster, "Hout"=w653:u64)  [unwired: 1 out]
        n381 = call "SCGetImageSize.vi"("Handle"=w653, "error in (no error)"=w654) -> ("Hout"=w652:u64, "error out"=w636:errorcluster, "Horizontal size"=w641:i32, "Vertical size"=w640:i32)  [unwired: 2 out]
        n382 = Greater?(x=w641, y=w640) -> (0:w642:bool)
        n383 = Initialize Array(u16 0 ("dimension size"), w640, w641) -> (w634:u16[][])
        n384 = call "SCRun.vi"("error in (no error)"=w636, "Run mode"=0, "Handle"=w652) -> ("error out"=w649:errorcluster, "Hout"=w648:u64)  [unwired: 1 out]
        n385 = Select(t=w641, s=w642, f=w640) -> (s? t:f=w639:i32)
        n386 = property on="mainimg" class="IntGraph (strict)"("XScale.Maximum"=w639, "YScale.Maximum"=w639) -> ()  [unwired: 2 in, 2 out]
      }
      frame "release" {
        n387 = Dequeue Element(queue=w680) -> (queue out=w667:refnum<queue>)  [unwired: 2 in, 3 out]
        n388 = flat-sequence {
          tunnel: w678 -> [w682]
          tunnel: [w681] -> w675
          tunnel: [w684] -> w676
          tunnel: w675 -> [w684]
          frame #0 {
            n389 = call "SCCloseBoard.vi"("Handle"=w682) -> ("error out"=w681:errorcluster)  [unwired: 1 in, 2 out]
          }
          frame #1 {
            n390 = local write "cam_con?"(FALSE ("cam_con?")) -> ()
          }
        }
        n391 = Enqueue Element(queue=w667, element="suspend") -> ()  [unwired: 2 in, 3 out]
        n392 = call <vilib>:"DAQmx Clear Task.vi"("task in"=w671) -> ()  [unwired: 14 in, 1 out]
      }
      frame "close" {
        n393 = Release Queue(queue=w693) -> ()  [unwired: 2 in, 3 out]
      }
      frame "idle", Default {
        n394 = call "grabimg.vi"("array in"=w734, "error in"=w740, "Hin"=w741) -> ("error out"=w739:errorcluster, "imgdata"=w737:i32[][], "Hout"=w738:u64)  [unwired: 6 in]
        n395 = local read "lower threshold"() -> (w732:i32)
        n396 = case shown="False" "cam_dark?" {
          tunnel: w743 -> [_ w766]
          tunnel: [w763 w765] -> w733
          tunnel: w737 -> [w763 w764]
          frame False {
          }
          frame True {
            n397 = Subtract(x=w764, y=w766) -> (x-y=w765:dbl[][])
          }
        }
        n398 = call "filtr_b.vi"("threshold"=w732, "input array"=w733) -> ("output array"=w724:dbl[][])  [unwired: 9 in]
        n399 = call <vilib>:"High Resolution Relative Seconds.vi"() -> ("relative seconds"=w748:dbl)
        n400 = Subtract(x=w748, y=w747) -> (x-y=w746:dbl)
        n401 = Array Size(array=w724) -> (size(s)=w723:i32[])
        n402 = Reciprocal(x=w746) -> (1/x=→"cam_fps":dbl)
        n403 = Index Array(array=w723) -> (element #1=w718:i32, element #2=w717:i32)  [unwired: 2 in]
        n404 = Subtract(x=w709, y=w708) -> (x-y=w707:i32)
        n405 = Less Or Equal?(x="pics2avg", y=w707) -> (x <= y?=w730:bool)
        n406 = And(x="reset every n pics", y=w730) -> (x .and. y?=w728:bool)
        n407 = Not(x=w728) -> (.not. x?=w727:bool)
        n408 = call-poly <vilib>:"Ramp Pattern.vi"("start"=0.0, "end"=w718, "samples"=w718) -> ("Ramp Pattern"=w713:dbl[])  [unwired: 7 in, 1 out]
        n409 = call-poly <vilib>:"Ramp Pattern.vi"("start"=0.0, "end"=w717, "samples"=w717) -> ("Ramp Pattern"=w714:dbl[])  [unwired: 7 in, 1 out]
        n410 = property on="mainimg" class="IntGraph (strict)"() -> ("CrsrLis"=w706:T4)  [unwired: 2 in, 2 out]
        n411 = And(x="cam_liveavg", y=w727) -> (x .and. y?=w725:bool)
        n412 = case shown="False" w725 {
          tunnel: w724 -> [w753 w759]
          tunnel: [w753 w756] -> w701
          tunnel: w736 -> [_ w761]
          tunnel: w709 -> [w754 _]
          tunnel: [w754 w762] -> w735
          tunnel: w708 -> [_ w762]
          tunnel: w707 -> [_ w755]
          frame False {
          }
          frame True {
            n413 = Multiply(x=w761, y=w755) -> (x*y=w760:dbl[][])
            n414 = Increment(x=w755) -> (x+1=w757:i32)
            n415 = Add(x=w760, y=w759) -> (x+y=w758:dbl[][])
            n416 = Divide(x=w758, y=w757) -> (x/y=w756:dbl[][])
          }
        }
        "mainimg" <- w701
        n417 = Index Array(array=w706) -> (element #1=w704:T6, element #2=w705:T6)  [unwired: 2 in]
        n418 = Unbundle By Name(w704) -> ("Position.X"=w698:dbl, "Position.Y"=w700:dbl)
        n419 = Unbundle By Name(w705) -> ("Position.X"=w702:dbl, "Position.Y"=w703:dbl)
        n420 = Array Max & Min(array=w701) -> (max value=→"max":dbl)  [unwired: 3 out]
        n421 = Subtract(x=w703, y=w700) -> (x-y=w699:dbl)
        n422 = Subtract(x=w702, y=w698) -> (x-y=w697:dbl)
        n423 = Array Subset(array=w701, index (row)=w700, length (row)=w699) -> (w712:dbl[][])  [unwired: 2 in]
        n424 = Array Subset(array=w701, index (col)=w698, length (col)=w697) -> (w710:dbl[][])  [unwired: 2 in]
        n425 = Array Subset(array=w701, index (row)=w700, length (row)=w699, index (col)=w698, length (col)=w697) -> (w696:dbl[][])
        n426 = Transpose 2D Array(2D array=w712) -> (transposed array=w711:dbl[][])
        n427 = Add Array Elements(numeric array=w696) -> (sum=→"sum" →"Waveform Chart":dbl)
        n428 = for {
          tunnel: w710 -> [w750] mode=indexing
          tunnel: [w749] -> w720 mode=indexing
          n429 = Add Array Elements(numeric array=w750) -> (sum=w749:dbl)
        }
        n430 = for {
          tunnel: w711 -> [w752] mode=indexing
          tunnel: [w751] -> w719 mode=indexing
          n431 = Add Array Elements(numeric array=w752) -> (sum=w751:dbl)
        }
        n432 = Bundle("Ramp Pattern"=w714, w719) -> (→"G2 X":cluster{"Ramp Pattern":dbl[], dbl[]})  [unwired: 1 in]
        n433 = Bundle(w720, "Ramp Pattern"=w713) -> (→"G2 Y":cluster{dbl[], "Ramp Pattern":dbl[]})  [unwired: 1 in]
      }
      frame "dark" {
        n434 = Dequeue Element(queue=w781) -> ()  [unwired: 2 in, 4 out]
        n435 = Array Size(array=w778) -> (size(s)=w777:i32[])
        n436 = Index Array(array=w777) -> (element #1=w776:i32, element #2=w775:i32)  [unwired: 2 in]
        n437 = Initialize Array(0.0 ("element"), w776, w775) -> (w773:dbl[][])
        n438 = for {
          N: "dark avg" -> [_]
          tunnel: w783 -> [w791]
          tunnel: w782 -> [w790]
          tunnel: [w789] -> w780
          tunnel: w778 -> [w788]
          tunnel: [w787] -> w779
          shift-right: [w784] -> w771
          shift-left: w773 -> [w785]
          n439 = call "grabimg.vi"("array in"=w788, "error in"=w790, "Hin"=w791) -> ("error out"=w789:errorcluster, "imgdata"=w786:i32[][], "Hout"=w787:u64)  [unwired: 6 in]
          n440 = Add(x=w786, y=w785) -> (x+y=w784:dbl[][])
        }
        n441 = Divide(x=w771, y="dark avg") -> (x/y=w772:dbl[][])
      }
      frame "snap" {
        n442 = Dequeue Element(queue=w811) -> ()  [unwired: 2 in, 4 out]
        n443 = local read "cam_dark?"() -> (w810:bool)
        n444 = local read "cam_avgs"() -> (w805:i32)
        n445 = To Double Precision Float(number=w796) -> (double precision float=w795:dbl[][])
        n446 = Equal To 0?(x="aq.mode") -> (x = 0?=w798:bool)
        n447 = Get Date/Time In Seconds() -> (seconds since 1Jan1904=w801:timestamp)
        n448 = for {
          N: w805 -> [w823]
          shift-right: [w840] -> w806
          shift-left: w808 -> [w842]
          shift-right: [w828] -> w804
          shift-left: w807 -> [w841]
          tunnel: w810 -> [w838]
          tunnel: w809 -> [w837]
          tunnel: w796 -> [w836]
          tunnel: w801 -> [w832]
          tunnel: w798 -> [w816]
          shift-right: [w824] -> w792
          shift-left: w795 -> [w825]
          shift-right: [w814] -> w793
          shift-left: w794 -> [w814]
          i -> [w812]
          stop <- "abort acq." stop-if-true
          n449 = call "grabimg.vi"("array in"=w836, "error in"=w841, "Hin"=w842) -> ("error out"=w828:errorcluster, "imgdata"=w839:i32[][], "Hout"=w840:u64)  [unwired: 6 in]
          n450 = local read "lower threshold"() -> (w819:i32)
          n451 = Increment(x=w812) -> (x+1=w821:i32)
          "acq. imgs" <- w821
          n452 = Get Date/Time In Seconds() -> (seconds since 1Jan1904=w835:timestamp)
          n453 = case shown="True" w838 {
            tunnel: w839 -> [w864 w867]
            tunnel: w837 -> [_ w866]
            tunnel: [w864 w865] -> w818
            frame False {
            }
            frame True {
              n454 = Subtract(x=w867, y=w866) -> (x-y=w865:dbl[][])
            }
          }
          n455 = Divide(x=w821, y=w823) -> (x/y=→"snap_prog":dbl)
          n456 = Subtract(x=w835, y=w832) -> (x-y=w834:dbl)
          n457 = call "filtr_b.vi"("threshold"=w819, "input array"=w818) -> ("output array"=w817:dbl[][])  [unwired: 9 in]
          n458 = Divide(x=w834, y=w812) -> (x/y=w830:dbl)
          n459 = Multiply(x=w830, y=w823) -> (x*y=w833:dbl)
          n460 = Reciprocal(x=w830) -> (1/x=w829:dbl)
          n461 = case shown="True" "count?" {
            tunnel: w817 -> [w855 w857]
            tunnel: "e-size" -> [_ w859]
            tunnel: w819 -> [_ w858]
            tunnel: [w855 w856] -> w815
            frame False {
            }
            frame True {
              n462 = Array Size(array=w857) -> (size(s)=w861:i32[])
              n463 = call "findr.vi"("thresh"=w858, "esize"=w859, "inp array"=w857) -> ("locs"=w860:i32[][])  [unwired: 8 in]
              n464 = Index Array(array=w861) -> (element #1=w863:i32, element #2=w862:i32)  [unwired: 2 in]
              n465 = call "drawe.vi"("Ysize"=w863, "Xsize"=w862, "pos array"=w860) -> ("img out"=w856:i32[][])  [unwired: 8 in]
            }
          }
          n466 = Add(x=w833, y=w832) -> (x+y=→"ETA":timestamp)
          n467 = local write "cam_fps"(w829) -> ()
          n468 = local write "mainimg"(w817) -> ()
          n469 = case shown="True" w816 {
            tunnel: w815 -> [w845 w853]
            tunnel: w825 -> [w847 w852]
            tunnel: [w846 w850] -> w824
            tunnel: [w844 w849] -> w813
            tunnel: w812 -> [w843 w848]
            frame False {
              n470 = Add(x=w845, y=w847) -> (x+y=w846:dbl[][])
              n471 = Increment(x=w843) -> (x+1=w844:i32)
            }
            frame True {
              n472 = Multiply(x=w852, y=w848) -> (x*y=w854:dbl[][])
              n473 = Increment(x=w848) -> (x+1=w849:i32)
              n474 = Add(x=w853, y=w854) -> (x+y=w851:dbl[][])
              n475 = Divide(x=w851, y=w849) -> (x/y=w850:dbl[][])
            }
          }
          "Pics L" <- w813
          n476 = local write "sideimg"(w824) -> ()
        }
        n477 = Enqueue Element(queue=w800, element=w792, error in (no error)=w804) -> (error out=w797:errorcluster)  [unwired: 1 in, 2 out]
      }
      frame "suspend" {
        n478 = Dequeue Element(queue=w876) -> ()  [unwired: 2 in, 4 out]
      }
    }
    "cam_error" <- w594
  }
  n479 = while {
    tunnel: w4 -> [w885]
    shift-right: [w882] -> _
    shift-left: _ -> [w883]
    tunnel: w3 -> [w881]
    shift-right: [w880] -> _
    shift-left: _ -> [w879]
    shift-right: [w877] -> _
    shift-left: _ -> [w878]
    stop <- w884 stop-if-true
    # "mirr"
    n480 = Preview Queue Element(queue=w885, timeout in ms (-1)=w883) -> (queue out=w888:refnum<queue>, element=w889:string)  [unwired: 1 in, 2 out]
    n481 = Match Pattern(string=w889, regular expression=":") -> (before substring=w887:string, after substring=w886:string)  [unwired: 1 in, 2 out]
    n482 = case shown="\"abs\"" w887 {
      tunnel: w888 -> [w924 w934 w949 w953 w956 w961 _]
      tunnel: w886 -> [w918 w935 _ _ _ _ _]
      tunnel: [_ _ _ TRUE _ _ _] -> w884
      tunnel: [_ _ _ _ -1 _ _] -> w882
      tunnel: w881 -> [w891 _ _ _ _ _ _]
      tunnel: [w910 w931 refnum<visa-resource-name> refnum ("VISA resource name out") w951 w955 w960 w966] -> w880
      tunnel: w879 -> [w923 w933 w948 w951 w955 _ w970]
      tunnel: [w895 w930 w947 w950 w954 w959 w965] -> w877
      tunnel: w878 -> [w922 w932 _ w950 w954 _ w969]
      frame "abs" {
        w906 = u8 20 items=["Echo"=55, "Home"=1, "Move Absolute"=20, "Move Relative"=21, "Move at Constant Speed"=22, "Renumber"=2, "Restore Settings"=36, "Stop"=23] ("Command")
        w921 = u8 20 items=["Echo"=55, "Home"=1, "Move Absolute"=20, "Move Relative"=21, "Move at Constant Speed"=22, "Renumber"=2, "Restore Settings"=36, "Stop"=23] ("Command")
        n483 = Dequeue Element(queue=w924) -> ()  [unwired: 2 in, 4 out]
        n484 = Match Pattern(string=w918, regular expression=":") -> (before substring=w908:string, after substring=w894:string)  [unwired: 1 in, 2 out]
        n485 = Equal?(x=w894, y="wait") -> (x = y?=w892:bool)
        n486 = Scan From String(format string="%g_%g", input string=w908) -> (output 1=w903:dbl, output 2=w902:dbl)  [unwired: 4 in, 3 out]
        n487 = local read "mirr_X#"() -> (w905:u8)
        n488 = Bundle("mirr_X#"=w905, "Command"=w921, w903, "Response Count"=1) -> (w917:T7)  [unwired: 1 in]
        n489 = local read "mirr_Y#"() -> (w904:u8)
        n490 = call "Request Command.vi"("error in (no error)"=w922, "Request"=w917, "VISA resource name"=w923) -> ("error out"=w899:errorcluster, "VISA resource name out"=w900:refnum<visa-resource-name>)  [unwired: 5 in, 2 out]
        n491 = Bundle("mirr_Y#"=w904, "Command"=w906, w902, "Response Count"=1) -> (w901:T8)  [unwired: 1 in]
        n492 = call "Request Command.vi"("error in (no error)"=w899, "Request"=w901, "VISA resource name"=w900) -> ("error out"=w897:errorcluster, "VISA resource name out"=w898:refnum<visa-resource-name>)  [unwired: 5 in, 2 out]
        n493 = local read "mirr_X#"() -> (w915:u8)
        n494 = call "zaber_readpos.vi"("error in (no error)"=w897, "axis"=w915, "VISA in"=w898) -> ("error out"=w911:errorcluster, "position"=w916:i32, "VISA out"=w912:refnum<visa-resource-name>)  [unwired: 6 in]
        n495 = local read "mirr_Y#"() -> (w913:u8)
        n496 = local write "mirr_posX"(w916) -> ()
        n497 = call "zaber_readpos.vi"("error in (no error)"=w911, "axis"=w913, "VISA in"=w912) -> ("error out"=w896:errorcluster, "position"=w914:i32, "VISA out"=w910:refnum<visa-resource-name>)  [unwired: 6 in]
        n498 = local write "mirr_posY"(w914) -> ()
        n499 = case shown="True" w892 {
          tunnel: w896 -> [w925 w929]
          tunnel: [w925 w928] -> w895
          tunnel: w891 -> [_ w927]
          frame False {
          }
          frame True {
            n500 = Send Notification(notification=TRUE, notifier=w927, error in (no error)=w929) -> (error out=w928:errorcluster)  [unwired: 1 out]
          }
        }
      }
      frame "rel" {
        w938 = u8 21 items=["Echo"=55, "Home"=1, "Move Absolute"=20, "Move Relative"=21, "Move at Constant Speed"=22, "Renumber"=2, "Restore Settings"=36, "Stop"=23] ("Command")
        n501 = Dequeue Element(queue=w934) -> ()  [unwired: 2 in, 4 out]
        n502 = Match Pattern(string=w935, regular expression=":") -> (before substring=w940:string, after substring=w939:string)  [unwired: 1 in, 2 out]
        n503 = Decimal String To Number(string=w940) -> (number=w942:i32)  [unwired: 2 in, 1 out]
        n504 = Decimal String To Number(string=w939) -> (number=w943:i32)  [unwired: 2 in, 1 out]
        n505 = Bundle(w942, "Command"=w938, w943, "Response Count"=1) -> (w936:T9)  [unwired: 1 in]
        n506 = call "Request Command.vi"("error in (no error)"=w932, "Request"=w936, "VISA resource name"=w933) -> ("error out"=w930:errorcluster, "VISA resource name out"=w931:refnum<visa-resource-name>)  [unwired: 5 in, 2 out]
      }
      frame "release" {
        n507 = Dequeue Element(queue=w949) -> (queue out=w945:refnum<queue>)  [unwired: 2 in, 3 out]
        n508 = Enqueue Element(queue=w945, element="suspend") -> ()  [unwired: 2 in, 3 out]
        n509 = call "Close.vi"("VISA resource name"=w948) -> ("error out"=w947:errorcluster)  [unwired: 9 in, 1 out]
      }
      frame "close" {
        n510 = Release Queue(queue=w953) -> ()  [unwired: 2 in, 3 out]
      }
      frame "suspend" {
        n511 = Dequeue Element(queue=w956) -> ()  [unwired: 2 in, 4 out]
      }
      frame "init" {
        n512 = Dequeue Element(queue=w961) -> ()  [unwired: 2 in, 4 out]
        n513 = call "Initialize.vi"("VISA resource name"="mirr_VISA") -> ("error out"=w959:errorcluster, "VISA resource name out"=w960:refnum<visa-resource-name>)  [unwired: 8 in, 1 out]
      }
      frame "idle", Default {
        n514 = local read "mirr_X#"() -> (w971:u8)
        n515 = call "zaber_readpos.vi"("error in (no error)"=w969, "axis"=w971, "VISA in"=w970) -> ("error out"=w967:errorcluster, "position"=→"mirr_posX":i32, "VISA out"=w968:refnum<visa-resource-name>)  [unwired: 6 in]
        n516 = local read "mirr_Y#"() -> (w964:u8)
        n517 = call "zaber_readpos.vi"("error in (no error)"=w967, "axis"=w964, "VISA in"=w968) -> ("error out"=w965:errorcluster, "position"=→"mirr_posY":i32, "VISA out"=w966:refnum<visa-resource-name>)  [unwired: 6 in]
      }
    }
    "mirr_Error" <- w877
  }
  n518 = while {
    tunnel: w13 -> [w980]
    shift-right: [w978] -> _
    shift-left: _ -> [w976]
    shift-right: [w977] -> _
    shift-left: _ -> [w975]
    shift-right: [w973] -> _
    shift-left: 0 -> [w974]
    tunnel: w3 -> [w972]
    stop <- w979 stop-if-true
    # "ESP"
    n519 = Preview Queue Element(queue=w980, timeout in ms (-1)=w974) -> (queue out=w983:refnum<queue>, element=w984:string)  [unwired: 1 in, 2 out]
    n520 = Match Pattern(string=w984, regular expression=":") -> (before substring=w982:string, after substring=w981:string)  [unwired: 1 in, 2 out]
    n521 = case shown="\"abs\"" w982 {
      tunnel: w983 -> [_ w995 w1013 w1054 w1057 w1064 w1069]
      tunnel: w981 -> [_ w1000 w1020 _ _ _ _]
      tunnel: [_ _ _ _ _ TRUE _] -> w979
      tunnel: [w987 w1002 w1014 w1052 refnum<visa-resource-name> refnum ("VISA resource name out") w1061 w1068] -> w978
      tunnel: [w986 w1003 w1012 w1051 w1059 w1062 w1067] -> w977
      tunnel: w976 -> [w991 w1005 w1018 w1052 w1060 w1061 _]
      tunnel: w975 -> [w990 w1004 w1019 w1051 _ w1062 _]
      tunnel: [_ _ _ -1 _ _ _] -> w973
      tunnel: w972 -> [_ _ w1006 _ _ _ _]
      frame "idle", Default {
        n522 = local read "ESP Axis"() -> (w988:i32)
        n523 = local read "ESP_t0"() -> (w994:dbl)
        n524 = call "Read Actual Position.vi"("error in (no error)"=w990, "Axis (1)"=w988, "VISA resource name"=w991) -> ("error out"=w986:errorcluster, "Position (units)"=w989:dbl, "VISA resource name out"=w987:refnum<visa-resource-name>)  [unwired: 2 in]
        "ESP_pos" <- w989
        n525 = call "mm2time.vi"("fs?"=TRUE, "Offset (mm)"=w994, "distance (mm)"=w989) -> ("time in fs/ps seconds"=→"ESP_delay":dbl)
      }
      frame "rel" {
        n526 = Match Pattern(string=w1000, regular expression=":") -> (before substring=w999:string, after substring=w998:string)  [unwired: 1 in, 2 out]
        n527 = Dequeue Element(queue=w995) -> ()  [unwired: 2 in, 4 out]
        n528 = Decimal String To Number(string=w999) -> (number=w997:i32)  [unwired: 2 in, 1 out]
        n529 = Fract/Exp String To Number(string=w998) -> (number=w996:dbl)  [unwired: 3 in, 1 out]
        n530 = call "Move Relative.vi"("error in (no error)"=w1004, "Position (0 units)"=w996, "Axis (1)"=w997, "VISA resource name"=w1005) -> ("error out"=w1003:errorcluster, "VISA resource name out"=w1002:refnum<visa-resource-name>)  [unwired: 2 in]
      }
      frame "abs" {
        n531 = Dequeue Element(queue=w1013) -> ()  [unwired: 2 in, 4 out]
        n532 = Match Pattern(string=w1020, regular expression=":") -> (before substring=w1021:string, after substring=w1010:string)  [unwired: 1 in, 2 out]
        n533 = Match Pattern(string=w1010, regular expression=":") -> (before substring=w1009:string, after substring=w1008:string)  [unwired: 1 in, 2 out]
        n534 = Decimal String To Number(string=w1021) -> (number=w1017:i32)  [unwired: 2 in, 1 out]
        n535 = Fract/Exp String To Number(string=w1009) -> (number=w1007:dbl)  [unwired: 3 in, 1 out]
        n536 = call "Move Absolute.vi"("error in (no error)"=w1019, "Position (0 units)"=w1007, "Axis (1)"=w1017, "VISA resource name"=w1018) -> ("error out"=w1015:errorcluster, "VISA resource name out"=w1016:refnum<visa-resource-name>)  [unwired: 2 in]
        n537 = case shown="\"wait\"" w1008 {
          tunnel: w1017 -> [_ w1039]
          tunnel: w1016 -> [w1024 w1041]
          tunnel: w1015 -> [w1023 w1040]
          tunnel: [w1024 w1027] -> w1014
          tunnel: [w1023 w1036] -> w1012
          tunnel: w1006 -> [_ w1035]
          frame "", Default {
          }
          frame "wait" {
            n538 = while {
              tunnel: w1039 -> [w1050]
              shift-right: [w1047] -> w1038
              shift-left: w1041 -> [w1049]
              shift-right: [w1046] -> w1037
              shift-left: w1040 -> [w1048]
              stop <- w1045 stop-if-true
              n539 = call "Get Axis Motion Status.vi"("error in (no error)"=w1048, "Axis (1)"=w1050, "VISA resource name"=w1049) -> ("error out"=w1046:errorcluster, "Motion Done"=w1045:bool, "VISA resource name out"=w1047:refnum<visa-resource-name>)  [unwired: 2 in]
            }
            n540 = flat-sequence {
              tunnel: w1038 -> [w1044]
              tunnel: w1037 -> [w1043]
              tunnel: [w1044] -> w1030
              tunnel: [w1043] -> w1029
              frame #0 {
                n541 = Wait (ms)(milliseconds to wait=u32 1000) -> ()  [unwired: 1 out]
              }
            }
            n542 = local read "ESP Axis"() -> (w1031:i32)
            n543 = local read "ESP_t0"() -> (w1033:dbl)
            n544 = call "Read Actual Position.vi"("error in (no error)"=w1029, "Axis (1)"=w1031, "VISA resource name"=w1030) -> ("error out"=w1028:errorcluster, "Position (units)"=w1025:dbl, "VISA resource name out"=w1027:refnum<visa-resource-name>)  [unwired: 2 in]
            n545 = call "mm2time.vi"("fs?"=TRUE, "Offset (mm)"=w1033, "distance (mm)"=w1025) -> ("time in fs/ps seconds"=w1026:dbl)
            n546 = local write "ESP_pos"(w1025) -> ()
            n547 = local write "ESP_delay"(w1026) -> ()
            n548 = Send Notification(notification=TRUE, notifier=w1035, error in (no error)=w1028) -> (error out=w1036:errorcluster)  [unwired: 1 out]
          }
        }
      }
      frame "suspend" {
        n549 = Dequeue Element(queue=w1054) -> ()  [unwired: 2 in, 4 out]
      }
      frame "release" {
        n550 = Dequeue Element(queue=w1057) -> (queue out=w1055:refnum<queue>)  [unwired: 2 in, 3 out]
        n551 = call "Close.vi"("VISA resource name"=w1060) -> ("error out"=w1059:errorcluster)  [unwired: 10 in]
        n552 = Enqueue Element(queue=w1055, element="suspend") -> ()  [unwired: 2 in, 3 out]
      }
      frame "close" {
        n553 = Release Queue(queue=w1064) -> ()  [unwired: 2 in, 3 out]
      }
      frame "init" {
        n554 = Dequeue Element(queue=w1069) -> ()  [unwired: 2 in, 4 out]
        n555 = flat-sequence {
          tunnel: [w1072] -> w1066
          tunnel: [w1071] -> w1065
          tunnel: [w1076] -> w1067
          tunnel: [w1077] -> w1068
          tunnel: w1066 -> [w1077]
          tunnel: w1065 -> [w1076]
          frame #0 {
            n556 = local write "ESP_con?"(FALSE ("ESP_con?")) -> ()
          }
          frame #1 {
            n557 = call "Initialize.vi"("VISA resource name"="ESP301 VISA", "Serial Link (RS232)"=enum16{"RS232", "USB"}."USB") -> ("VISA resource name out"=w1072:refnum<visa-resource-name>, "error out"=w1071:errorcluster)  [unwired: 7 in]
          }
          frame #2 {
            n558 = local write "ESP_con?"(TRUE ("ESP_con?")) -> ()
          }
        }
      }
    }
    "error out" <- w977
  }
  n559 = while {
    tunnel: w12 -> [w1086]
    shift-right: [w1084] -> _
    shift-left: _ -> [w1082]
    shift-right: [w1083] -> _
    shift-left: _ -> [w1081]
    shift-right: [w1079] -> _
    shift-left: 0 -> [w1080]
    tunnel: w3 -> [w1078]
    stop <- w1085 stop-if-true
    # "manip"
    n560 = Preview Queue Element(queue=w1086, timeout in ms (-1)=w1080) -> (queue out=w1089:refnum<queue>, element=w1090:string)  [unwired: 1 in, 2 out]
    n561 = Match Pattern(string=w1090, regular expression=":") -> (before substring=w1088:string, after substring=w1087:string)  [unwired: 1 in, 2 out]
    n562 = case shown="\"idle\", Default" w1088 {
      tunnel: w1089 -> [_ w1102 w1129 w1170 w1208 w1214 w1223 w1228]
      tunnel: w1087 -> [_ _ w1116 w1169 _ _ _ _]
      tunnel: [_ _ _ _ _ _ TRUE _] -> w1085
      tunnel: [w1096 w1104 w1108 w1167 w1210 refnum<k5> refnum ("gateway_connection out") w1221 w1227] -> w1084
      tunnel: [w1095 w1103 w1110 w1166 w1209 w1216 w1220 w1226] -> w1083
      tunnel: w1082 -> [w1098 w1106 w1132 w1160 w1210 w1218 w1221 _]
      tunnel: w1081 -> [w1097 w1105 w1131 w1161 w1209 _ w1220 _]
      tunnel: [_ _ _ _ -1 _ _ _] -> w1079
      tunnel: w1078 -> [_ _ w1107 w1163 _ _ _ _]
      frame "idle", Default {
        n563 = call "sp_manip_get_axis_status.vi"("error in"=w1097, "gateway_connection"=w1098) -> ("error out"=w1095:errorcluster, "axis_out"=w1094:T10, "gateway_connection out"=w1096:refnum<k5>)  [unwired: 5 in, 2 out]
        n564 = for {
          tunnel: w1094 -> [w1101] mode=indexing
          tunnel: [w1100] -> w1093 mode=indexing
          tunnel: [w1099] -> w1092 mode=indexing
          n565 = Unbundle By Name(w1101) -> ("Axis_Position"=w1100:dbl, "moving"=w1099:bool)
        }
        "moving?" <- w1092
        n566 = local write "pos"(w1093) -> ()
      }
      frame "stop" {
        n567 = Dequeue Element(queue=w1102) -> ()  [unwired: 2 in, 4 out]
        n568 = call "sp_manip_abort.vi"("error in"=w1105, "gateway_connection"=w1106) -> ("error out"=w1103:errorcluster, "gateway_connection out"=w1104:refnum<k5>)  [unwired: 6 in, 2 out]
      }
      frame "rel" {
        n569 = Dequeue Element(queue=w1129) -> ()  [unwired: 2 in, 4 out]
        n570 = Match Pattern(string=w1116, regular expression=":") -> (before substring=w1115:string, after substring=w1114:string)  [unwired: 1 in, 2 out]
        n571 = Equal?(x=w1114, y="wait") -> (x = y?=w1112:bool)
        n572 = call "sp_manip_get_axis_status.vi"("error in"=w1131, "gateway_connection"=w1132) -> ("error out"=w1134:errorcluster, "axis_out"=w1121:T10, "gateway_connection out"=w1133:refnum<k5>)  [unwired: 5 in, 2 out]
        n573 = Scan From String(format string="%g_%g_%g_%g_%g_%g", input string=w1115) -> (output 1=w1128:dbl, output 2=w1127:dbl, output 3=w1126:dbl, output 4=w1125:dbl, output 5=w1124:dbl, output 6=w1123:dbl)  [unwired: 8 in, 3 out]
        n574 = for {
          tunnel: w1121 -> [w1155] mode=indexing
          tunnel: [w1154] -> w1119 mode=indexing
          tunnel: [w1153] -> w1120 mode=indexing
          n575 = Unbundle By Name(w1155) -> ("Axis_Name"=w1154:string, "Axis_Position"=w1153:dbl)
        }
        n576 = Build Array(w1128, w1127, w1126, w1125, w1124, w1123) -> (w1122:dbl[])
        n577 = Add(x=w1120, y=w1122) -> (x+y=w1118:dbl[])
        n578 = call "sp_manip_start_move.vi"("error in"=w1134, "target positions"=w1118, "axis names"=w1119, "gateway_connection"=w1133) -> ("error out"=w1111:errorcluster, "gateway_connection out"=w1109:refnum<k5>)  [unwired: 4 in, 2 out]
        n579 = case shown="True" w1112 {
          tunnel: w1111 -> [w1135 w1142]
          tunnel: [w1135 w1139] -> w1110
          tunnel: w1109 -> [w1136 w1143]
          tunnel: [w1136 w1141] -> w1108
          tunnel: w1107 -> [_ w1138]
          frame False {
          }
          frame True {
            n580 = while {
              tunnel: w1143 -> [w1147]
              tunnel: w1142 -> [w1146]
              tunnel: [w1145] -> w1141
              tunnel: [w1144] -> w1140
              stop <- w1148 continue-if-true
              n581 = call "sp_manip_get_axis_status.vi"("error in"=w1146, "gateway_connection"=w1147) -> ("error out"=w1144:errorcluster, "axis_out"=w1150:T10, "gateway_connection out"=w1145:refnum<k5>)  [unwired: 5 in, 2 out]
              n582 = for {
                tunnel: w1150 -> [w1152] mode=indexing
                tunnel: [w1151] -> w1149 mode=indexing
                n583 = Unbundle By Name(w1152) -> ("moving"=w1151:bool)
              }
              n584 = Or Array Elements(Boolean array=w1149) -> (logical OR=w1148:bool)
            }
            n585 = Send Notification(notification=TRUE, notifier=w1138, error in (no error)=w1140) -> (error out=w1139:errorcluster)  [unwired: 1 out]
          }
        }
      }
      frame "abs" {
        n586 = Dequeue Element(queue=w1170) -> ()  [unwired: 2 in, 4 out]
        n587 = call "sp_manip_get_axis_status.vi"("error in"=w1161, "gateway_connection"=w1160) -> ("error out"=w1156:errorcluster, "axis_out"=w1159:T10, "gateway_connection out"=w1157:refnum<k5>)  [unwired: 5 in, 2 out]
        n588 = Match Pattern(string=w1169, regular expression=":") -> (before substring=w1173:string, after substring=w1172:string)  [unwired: 1 in, 2 out]
        n589 = Equal?(x=w1172, y="wait") -> (x = y?=w1162:bool)
        n590 = for {
          tunnel: w1159 -> [w1183] mode=indexing
          tunnel: [w1182] -> w1158 mode=indexing
          n591 = Unbundle By Name(w1183) -> ("Axis_Name"=w1182:string)
        }
        n592 = Scan From String(format string="%g_%g_%g_%g_%g_%g", input string=w1173) -> (output 1=w1179:dbl, output 2=w1178:dbl, output 3=w1177:dbl, output 4=w1176:dbl, output 5=w1175:dbl, output 6=w1174:dbl)  [unwired: 8 in, 3 out]
        n593 = Build Array(w1179, w1178, w1177, w1176, w1175, w1174) -> (w1181:dbl[])
        n594 = call "sp_manip_start_move.vi"("error in"=w1156, "target positions"=w1181, "axis names"=w1158, "gateway_connection"=w1157) -> ("error out"=w1165:errorcluster, "gateway_connection out"=w1164:refnum<k5>)  [unwired: 4 in, 2 out]
        n595 = case shown="True" w1162 {
          tunnel: w1165 -> [w1184 w1195]
          tunnel: [w1184 w1194] -> w1166
          tunnel: w1164 -> [w1185 w1196]
          tunnel: [w1185 w1187] -> w1167
          tunnel: w1163 -> [_ w1193]
          frame False {
          }
          frame True {
            n596 = while {
              tunnel: w1196 -> [w1202]
              tunnel: w1195 -> [w1201]
              tunnel: [w1200] -> w1189
              tunnel: [w1199] -> w1188
              stop <- w1203 continue-if-true
              n597 = call "sp_manip_get_axis_status.vi"("error in"=w1201, "gateway_connection"=w1202) -> ("error out"=w1199:errorcluster, "axis_out"=w1205:T10, "gateway_connection out"=w1200:refnum<k5>)  [unwired: 5 in, 2 out]
              n598 = for {
                tunnel: w1205 -> [w1207] mode=indexing
                tunnel: [w1206] -> w1204 mode=indexing
                n599 = Unbundle By Name(w1207) -> ("moving"=w1206:bool)
              }
              n600 = Or Array Elements(Boolean array=w1204) -> (logical OR=w1203:bool)
            }
            n601 = call "sp_manip_get_axis_status.vi"("error in"=w1188, "gateway_connection"=w1189) -> ("error out"=w1186:errorcluster, "axis_out"=w1191:T10, "gateway_connection out"=w1187:refnum<k5>)  [unwired: 5 in, 2 out]
            n602 = for {
              tunnel: w1191 -> [w1198] mode=indexing
              tunnel: [w1197] -> w1190 mode=indexing
              n603 = Unbundle By Name(w1198) -> ("Axis_Position"=w1197:dbl)
            }
            n604 = local write "pos"(w1190) -> ()
            n605 = Send Notification(notification=TRUE, notifier=w1193, error in (no error)=w1186) -> (error out=w1194:errorcluster)  [unwired: 1 out]
          }
        }
      }
      frame "suspend" {
        n606 = Dequeue Element(queue=w1208) -> ()  [unwired: 2 in, 4 out]
      }
      frame "release" {
        n607 = Dequeue Element(queue=w1214) -> (queue out=w1212:refnum<queue>)  [unwired: 2 in, 3 out]
        n608 = call "sp_manip_disconnect.vi"("gateway_connection"=w1218) -> ("error out"=w1217:errorcluster, "gateway_connection_out"=w1219:refnum<k5>)  [unwired: 7 in, 2 out]
        n609 = call "tcp_gateway_close_connection.vi"("error in"=w1217, "server_connection"=w1219) -> ("error out"=w1216:errorcluster)  [unwired: 5 in]
        n610 = Enqueue Element(queue=w1212, element="suspend") -> ()  [unwired: 2 in, 3 out]
      }
      frame "close" {
        n611 = Release Queue(queue=w1223) -> ()  [unwired: 2 in, 3 out]
      }
      frame "init" {
        n612 = Dequeue Element(queue=w1228) -> ()  [unwired: 2 in, 4 out]
        n613 = flat-sequence {
          tunnel: [w1231] -> w1225
          tunnel: [w1230] -> w1224
          tunnel: [w1241] -> w1226
          tunnel: [w1242] -> w1227
          tunnel: w1225 -> [w1242]
          tunnel: w1224 -> [w1241]
          frame #0 {
            n614 = local write "manip_con?"(FALSE ("manip_con?")) -> ()
          }
          frame #1 {
            n615 = call "tcp_gateway_open_connection.vi"() -> ("gateway_connection"=w1234:refnum<k5>, "error out"=w1233:errorcluster)  [unwired: 5 in, 3 out]
            n616 = call "sp_manip_connect.vi"("error in"=w1233, "gateway_connection"=w1234) -> ("error out"=w1230:errorcluster, "axis_out"=w1232:T10, "gateway_connection out"=w1231:refnum<k5>)  [unwired: 5 in, 2 out]
            n617 = for {
              tunnel: w1232 -> [w1239] mode=indexing
              tunnel: [w1238] -> w1235 mode=indexing
              tunnel: [w1237] -> w1236 mode=indexing
              n618 = Unbundle By Name(w1239) -> ("Axis_Name"=w1238:string, "Axis_Position"=w1237:dbl)
            }
            "axis" <- w1235
            "pos" <- w1236
            n619 = local write "dest"(w1236) -> ()
          }
          frame #2 {
            n620 = local write "manip_con?"(TRUE ("manip_con?")) -> ()
          }
        }
      }
    }
    "error out 2" <- w1083
  }
  n621 = while {
    tunnel: w11 -> [w1254]
    shift-right: [w1243] -> _
    shift-left: 0 -> [w1252]
    shift-right: [w1251] -> _
    shift-left: _ -> [w1250]
    shift-right: [w1249] -> _
    shift-left: _ -> [w1248]
    shift-right: [w1247] -> _
    shift-left: u32 0 ("pHandle") -> [w1246]
    tunnel: w9 -> [w1245]
    tunnel: w3 -> [w1244]
    stop <- w1253 stop-if-true
    # "phoib"
    n622 = Preview Queue Element(queue=w1254, timeout in ms (-1)=w1252) -> (queue out=w1257:refnum<queue>, element=w1258:string)  [unwired: 1 in, 2 out]
    n623 = Match Pattern(string=w1258, regular expression=":") -> (before substring=w1256:string, after substring=w1255:string)  [unwired: 1 in, 2 out]
    n624 = case shown="\"idle\", Default" w1256 {
      tunnel: w1257 -> [_ w1311 w1365 w1382 w1400 w1414 w1419 w1424]
      tunnel: w1255 -> [_ _ w1361 _ _ _ _ _]
      tunnel: [_ _ _ _ _ TRUE _ _] -> w1253
      tunnel: [w1268 w1313 w1330 w1385 w1398 w1412 w1418 w1421] -> w1251
      tunnel: w1250 -> [w1279 w1302 w1351 w1387 w1399 w1412 w1418 _]
      tunnel: [w1267 w1312 w1346 w1384 w1397 w1410 w1416 w1420] -> w1249
      tunnel: w1248 -> [w1277 w1301 _ w1386 _ w1410 w1416 _]
      tunnel: [w1265 w1299 w1329 w1383 w1396 w1411 w1417 w1423] -> w1247
      tunnel: w1246 -> [w1265 w1299 w1349 w1383 w1395 w1411 w1417 _]
      tunnel: w1245 -> [w1266 w1292 w1327 _ _ _ _ _]
      tunnel: w1244 -> [_ _ w1345 _ _ _ _ _]
      tunnel: [_ _ _ _ _ _ -1 _] -> w1243
      frame "idle", Default {
        n625 = call "SL2_AD_DLL_Phoibos_GetDeviceState.vi"("dll_path"=w1279, "pHandle_in"=w1265, "dev_type"=DEF_dev_type."devA (analyzer)", "error in"=w1277) -> ("path out"=w1264:path, "state"=→"state":T2, "error out"=w1263:errorcluster)  [unwired: 2 in]
        n626 = for {
          tunnel: w1265 -> [w1286]
          tunnel: w1266 -> [w1284] mode=indexing
          tunnel: [w1283] -> w1276 mode=indexing
          tunnel: [w1282] -> w1268
          shift-right: [w1281] -> w1267
          shift-left: w1263 -> [w1285]
          tunnel: w1264 -> [w1280]
          n627 = call "SL2_AD_DLL_Phoibos_GetVoltage.vi"("error in"=w1285, "voltage_name"=w1284, "pHandle"=w1286, "dll path in"=w1280) -> ("error out"=w1281:errorcluster, "value"=w1283:dbl, "dll path out"=w1282:path)  [unwired: 3 in]
        }
        n628 = Index Array(array=w1276) -> (element #1=→"phoib_I_1":dbl, element #2=→"phoib_I_2":dbl, element #3=→"phoib_I_3":dbl, element #4=→"phoib_I_4":dbl, element #5=→"phoib_I_5":dbl, element #6=→"phoib_I_6":dbl, element #7=→"phoib_I_7":dbl, element #8=→"phoib_I_8":dbl, element #9=→"phoib_I_9":dbl)  [unwired: 9 in]
      }
      frame "set" {
        n629 = Dequeue Element(queue=w1311) -> ()  [unwired: 2 in, 4 out]
        n630 = Multiply(x="ana_voltrange", y=13) -> (x*y=w1308:i32)
        n631 = Add(x="ana_mode", y=w1308) -> (x+y=w1305:i32)
        n632 = Index Array(array=u32[] [251749632, 251749633, 251749634, 251749635, 251749636, 251749637, 251749638, 251749639, 251749640, 251749641, 251749642, 251749643, 251749644, 251749645, 251749646, 251749647, 251749648, 251749649, 251749650, 251749651, 251749652, 251749653, 251749654, 251749655, 251749656, 251749657, 251749658, 251749659, 251749660, 251749661, 251749662, 251749663, 251749664, 251749665, 251749666, 251749667, 251749668, 251749669, 251749670, 251749671, 251749672, 251749673, 251749674, 251749675, 251749676, 251749677, 251749678, 251749679, 251749680, 251749681, 251749682, 251749683, 251749684, 251749685, 251749686, 251749687, 251749688, 251749689, 251749690, 251749691, 251749692, 251749693, 251749694, 251749695, 251749696] ("modeIDs"), index=w1305) -> (element=w1303:u32)
        n633 = Build Array("phoib_I_1s", "phoib_I_2s", "phoib_I_3s", "phoib_I_4s", "phoib_I_5s", "phoib_I_6s", "phoib_I_7s", "phoib_I_8s", "phoib_I_9s") -> (w1291:dbl[])
        n634 = call "SL2_AD_DLL_Phoibos_SetDeviceMode.vi"("pHandle"=w1299, "error in"=w1301, "value"=w1303, "dev_type"=DEF_dev_type."devA (analyzer)", "dll path in"=w1302) -> ("error out"=w1290:errorcluster, "dll path out"=w1300:path)  [unwired: 4 in]
        n635 = for {
          tunnel: w1299 -> [w1319]
          shift-right: [w1326] -> w1313
          shift-left: w1300 -> [w1323]
          tunnel: w1292 -> [w1318] mode=indexing
          tunnel: w1291 -> [w1317] mode=indexing
          shift-right: [w1325] -> w1312
          shift-left: w1290 -> [w1321]
          n636 = call "SL2_AD_DLL_Phoibos_GetVoltageRange.vi"("error in"=w1321, "voltage_name"=w1318, "pHandle"=w1319, "dll path in"=w1323) -> ("error out"=w1320:errorcluster, "min"=w1315:dbl, "max"=w1316:dbl, "dll path out"=w1322:path)  [unwired: 2 in]
          n637 = In Range and Coerce(upper limit=w1316, x=w1317, lower limit=w1315) -> (coerced(x)=w1314:dbl)  [unwired: 1 out]
          n638 = call "SL2_AD_DLL_Phoibos_SetVoltage.vi"("commit"=TRUE, "pHandle"=w1319, "error in"=w1320, "value"=w1314, "voltageName"=w1318, "dll path in"=w1322) -> ("error out"=w1325:errorcluster, "dll path out"=w1326:path)  [unwired: 3 in]
        }
      }
      frame "setsgl" {
        n639 = Dequeue Element(queue=w1365) -> ()  [unwired: 2 in, 4 out]
        n640 = Match Pattern(string=w1361, regular expression=":") -> (before substring=w1354:string, after substring=w1363:string)  [unwired: 1 in, 2 out]
        n641 = Equal?(x=w1363, y="wait") -> ()  [unwired: 1 out]
        n642 = Match Pattern(string=w1354, regular expression=":") -> (before substring=w1328:string, after substring=w1353:string)  [unwired: 1 in, 2 out]
        n643 = Fract/Exp String To Number(string=w1353) -> (number=w1352:dbl)  [unwired: 3 in, 1 out]
        n644 = call "SL2_AD_DLL_Phoibos_GetVoltageRange.vi"("voltage_name"=w1328, "pHandle"=w1349, "dll path in"=w1351) -> ("error out"=w1358:errorcluster, "min"=w1356:dbl, "max"=w1357:dbl, "dll path out"=w1359:path)  [unwired: 3 in]
        n645 = In Range and Coerce(upper limit=w1357, x=w1352, lower limit=w1356) -> (coerced(x)=w1347:dbl)  [unwired: 1 out]
        n646 = call "SL2_AD_DLL_Phoibos_SetVoltage.vi"("commit"=TRUE, "pHandle"=w1349, "error in"=w1358, "value"=w1347, "voltageName"=w1328, "dll path in"=w1359) -> ("error out"=w1348:errorcluster, "dll path out"=w1350:path)  [unwired: 3 in]
        n647 = while {
          tunnel: w1350 -> [w1381]
          tunnel: w1349 -> [w1375]
          tunnel: w1328 -> [w1380]
          tunnel: w1348 -> [w1379]
          tunnel: w1347 -> [w1378]
          tunnel: [w1375] -> w1329
          tunnel: [w1374] -> w1331
          tunnel: [w1373] -> w1333
          stop <- w1376 stop-if-true
          n648 = call "SL2_AD_DLL_Phoibos_GetVoltage.vi"("error in"=w1379, "voltage_name"=w1380, "pHandle"=w1375, "dll path in"=w1381) -> ("error out"=w1373:errorcluster, "value"=w1377:dbl, "dll path out"=w1374:path)  [unwired: 3 in]
          n649 = Equal?(x=w1378, y=w1377) -> (x = y?=w1376:bool)
        }
        n650 = for {
          tunnel: w1329 -> [w1372]
          tunnel: [w1370] -> w1334 mode=indexing
          tunnel: [w1369] -> w1330
          shift-right: [w1368] -> w1332
          shift-left: w1333 -> [w1371]
          tunnel: w1331 -> [w1367]
          tunnel: w1327 -> [w1366] mode=indexing
          n651 = call "SL2_AD_DLL_Phoibos_GetVoltage.vi"("error in"=w1371, "voltage_name"=w1366, "pHandle"=w1372, "dll path in"=w1367) -> ("error out"=w1368:errorcluster, "value"=w1370:dbl, "dll path out"=w1369:path)  [unwired: 3 in]
        }
        n652 = Index Array(array=w1334) -> (element #1=w1335:dbl, element #2=w1336:dbl, element #3=w1337:dbl, element #4=w1338:dbl, element #5=w1339:dbl, element #6=w1343:dbl, element #7=w1340:dbl, element #8=w1341:dbl, element #9=w1342:dbl)  [unwired: 9 in]
        n653 = local write "phoib_I_1"(w1335) -> ()
        n654 = local write "phoib_I_2"(w1336) -> ()
        n655 = local write "phoib_I_3"(w1337) -> ()
        n656 = local write "phoib_I_4"(w1338) -> ()
        n657 = local write "phoib_I_5"(w1339) -> ()
        n658 = local write "phoib_I_6"(w1343) -> ()
        n659 = local write "phoib_I_7"(w1340) -> ()
        n660 = local write "phoib_I_8"(w1341) -> ()
        n661 = local write "phoib_I_9"(w1342) -> ()
        n662 = Send Notification(notification=TRUE, notifier=w1345, error in (no error)=w1332) -> (error out=w1346:errorcluster)  [unwired: 1 out]
      }
      frame "standby" {
        w1388 = T2 0 items=["Off"=-1, "Standby"=0, "On"=1] ("state")
        n663 = Dequeue Element(queue=w1382) -> ()  [unwired: 2 in, 4 out]
        n664 = call "SL2_AD_DLL_Phoibos_SetDeviceState.vi"("pHandle_in"=w1383, "error in"=w1386, "state"=w1388, "dev_type"=DEF_dev_type."devA (analyzer)", "dll_path"=w1387) -> ("error out"=w1384:errorcluster, "path out"=w1385:path)  [unwired: 2 in]
      }
      frame "release" {
        n665 = Dequeue Element(queue=w1400) -> (queue out=w1390:refnum<queue>)  [unwired: 2 in, 3 out]
        n666 = flat-sequence {
          tunnel: w1399 -> [w1401]
          tunnel: w1395 -> [w1402]
          tunnel: [w1405] -> w1394
          tunnel: [w1404] -> w1393
          tunnel: [u32 0] -> w1392
          tunnel: [w1407] -> w1396
          tunnel: [w1408] -> w1397
          tunnel: [w1409] -> w1398
          tunnel: w1394 -> [w1409]
          tunnel: w1393 -> [w1408]
          tunnel: w1392 -> [w1407]
          frame #0 {
            n667 = call "SL2_AD_DLL_Phoibos_Shutdown.vi"("pHandle"=w1402, "dll path in"=w1401) -> ("error out"=w1404:errorcluster, "dll path out"=w1405:path)  [unwired: 4 in]
          }
          frame #1 {
            n668 = local write "phoib_con?"(FALSE ("phoib_con?")) -> ()
          }
        }
        n669 = Enqueue Element(queue=w1390, element="suspend") -> ()  [unwired: 2 in, 3 out]
      }
      frame "close" {
        n670 = Release Queue(queue=w1414) -> ()  [unwired: 2 in, 3 out]
      }
      frame "suspend" {
        n671 = Dequeue Element(queue=w1419) -> ()  [unwired: 2 in, 4 out]
      }
      frame "init" {
        n672 = Dequeue Element(queue=w1424) -> ()  [unwired: 2 in, 4 out]
        n673 = flat-sequence {
          tunnel: [w1431] -> w1422
          tunnel: [w1427] -> w1421
          tunnel: [w1426] -> w1420
          tunnel: [w1439] -> w1423
          tunnel: w1422 -> [w1439]
          frame #0 {
            n674 = local write "phoib_con?"(FALSE ("phoib_con?")) -> ()
          }
          frame #1 {
            w1430 = DEF_dev_type."devA (analyzer)" ("dev_type")
            n675 = call "GetSL2AD_VI_dllPath.vi"() -> ("error"=w1434:errorcluster, "Path"=w1435:path)  [unwired: 9 in, 1 out]
            n676 = call "SL2_AD_DLL_List_Devices.vi"("error in"=w1434, "dev_type"=w1430, "dll path in"=w1435) -> ("error out"=w1428:errorcluster, "devices"=w1437:string[], "dll path out"=w1429:path)  [unwired: 2 in]
            n677 = Index Array(array=w1437) -> (element=w1436:string)  [unwired: 1 in]
            n678 = call "SL2_AD_DLL_Phoibos_Initialize.vi"("error in"=w1428, "analyzerId"=w1436, "dll_path"=w1429) -> ("error out"=w1432:errorcluster, "pHandle"=w1431:u32, "path out"=w1433:path)  [unwired: 2 in]
            n679 = call "SL2_AD_DLL_Phoibos_ListDeviceModes.vi"("dll path in"=w1433, "dev_type"=w1430, "pHandle"=w1431, "error in"=w1432) -> ("dll path out"=w1427:path, "error out"=w1426:errorcluster)  [unwired: 1 in, 2 out]
          }
          frame #2 {
            n680 = local write "phoib_con?"(TRUE ("phoib_con?")) -> ()
          }
        }
      }
    }
    "phoib_error" <- w1249
  }
